vi "red_tweezers_interface.vi"() -> ()   [LabVIEW 2010]
doc: "This is the interface, the one VI which loads all the others. Run this one first.\n\n(the line below ensures settings are saved)\n[Red Tweezers Save Settings]"
uses:
  subvis/line_trapping.ctl
  subvis/spot.ctl
  <vilib>/userDefined/High Color/IMAQdx.ctl
  subvis/mouse_info.ctl
  subvis/selection_element.ctl
  subvis/red_tweezers_globals.vi
  subvis/red_tweezers_globals_INTERNAL_VOLATILE.vi
  <vilib>/Analysis/baseanly.llb/Real A x B.vi
  <vilib>/Analysis/NI_AALBase.lvlib
  <vilib>/vision/driver/NI_Vision_Acquisition_Software.lvlib
panel:
  out "# selected":i16
  out "Last Pattern":T1[](array[typedef]) {"Amplitude Correction" step=0.1; "Line Trapping"."Phase Gradient" step=0.05; "Line Trapping"."Vector"."x" step=1e-06 format="%#_6p"; "Line Trapping"."Vector"."y" step=1e-06 format="%#_6p"; "Line Trapping"."Vector"."z" step=1e-06 format="%#_6p"; "NA Position"."r" step=1e-06; "NA Position"."y" step=1e-06; "NA Position"."x" step=1e-06; "Position"."z" step=1e-06; "Position"."y" step=1e-06; "Position"."x" step=1e-06; "Phase" step=0.7753; "Intensity" step=0.1}
  out "Plugins":T3(array[cluster])=[{"Name"="ASI Stage", "Folder"=path "C:/Users/Richard Bowman/Dropbox/red_tweezers_1_4_rc4/plugins/ASI Stage.llb", "vi reference"=refnum, "Needs to be run"=TRUE, "Error"={"status"=FALSE, "code"=0, "source"=""}}, {"Name"="iTweezers", "Folder"=path "C:/Users/Richard Bowman/Dropbox/red_tweezers_1_4_rc4/plugins/iTweezers.llb", "vi reference"=refnum, "Needs to be run"=TRUE, "Error"={"status"=FALSE, "code"=0, "source"=""}}, {"Name"="MightexLED", "Folder"=path "C:/Users/Richard Bowman/Dropbox/red_tweezers_1_4_rc4/plugins/MightexLED.llb", "vi reference"=refnum, "Needs to be run"=TRUE, "Error"={"status"=FALSE, "code"=0, "source"=""}}]
  in  "Tab":T4(tab)
  out "spots selected":i32=4
  in  "lock aspect ratio":bool=TRUE
  in  "Size":cluster{"x":dbl, "y":dbl, "z":dbl} {"z" step=1e-06 format="%#_4p"; "y" step=1e-06 format="%#_4p"; "x" step=1e-06 format="%#_4p"}
  in  "Position":cluster{"x":dbl, "y":dbl, "z":dbl}={"x"=1e-06, "y"=-6.3e-06, "z"=0.0} {"z" step=1e-06 format="%#_4p"; "y" step=1e-06 format="%#_4p"; "x" step=1e-06 format="%#_4p"}
  in  "phase":dbl step=0.7753
  in  "Vortex Charge":i8
  in  "Intensity":dbl=1.0 step=0.1
  in  "add to selection":bool
  in  "random position":bool
  in  "new spot":bool
  in  "delete":bool
  in  "rotate":bool
  in  "Rotation Axis":u16(ring)=2 items=["Z", "X", "Y", "Custom"]
  in  "Angle (degrees)":dbl=2.0
  in  "Custom Axis":cluster{dbl, dbl, dbl}
  in  "Spot Shape":enum32{"Normal", "Line", "NA", "Mixed"}(tab)=enum."Mixed"
  in  "Line Trapping":T2 {"Phase Gradient" step=0.05; "Vector"."x" step=1e-06 format="%#_4p"; "Vector"."y" step=1e-06 format="%#_4p"; "Vector"."z" step=1e-06 format="%#_4p"}
  in  "Scale back aperture":dbl=1.1 step=0.1
  in  "Scale BA":bool
  in  "Position on back aperture":cluster{"x":dbl, "y":dbl}={"x"=-5.84327907697451e-18, "y"=0.0} {"y" step=0.1 format="%#_4p"; "x" step=0.1 format="%#_4p"}
  in  "Radius on back aperture":dbl=1.1 step=0.1
  in  "Generate":bool
  in  "Pattern":T5(tab)
  in  "Spots across centre":i32=5
  in  "Reference Array?":bool
  in  "Fraction of SLM":dbl=1.0
  in  "Spots across centre":i32=5
  in  "N":cluster{i32, i32}
  in  "spacing/m":dbl=2.0
  in  "Iterations":i32=10
  out "non-uniformity":dbl(slide)=0.031119223416512406 scale=0.0..0.2
  out "efficiency":dbl(slide)=0.8985936267644501 scale=0.0..1.0
  in  "Optimise":bool
  in  "Reset Phase/Amplitude":bool
  in  "Fall-off/m":dbl=0.00025 min=0.0 step=1e-06 format="%#_4p"
  in  "Abort Plugin":bool
  in  "Plugin:":u16(ring)=1 items=["ASI Stage", "iTweezers", "MightexLED"]
  in  "Save Video":bool
  in  "Global ROI (requires restart)":i32[](array[numeric])=[0, 0, 1280, 512]
  in  "Zoom":bool
  in  "Draw ROI":bool
  in  "Zoom to Fit":bool
  out "Image Information":string="640x480 1.93X 8-bit image 255    (0,0)"
  in  "Camera":T6
  out "Video Frame Rate":dbl(knob)=50.00000000000003 scale=0.0..100.0 scale format="%.1f"
  out "Interface Frame Rate":dbl(knob)=97.23240312927678 scale=0.0..100.0 scale format="%.1f"
  in  "stop":bool=TRUE
  out "Image":T7(plugin-control)
  # "The SLM can be used to shape spots; here you can restrict the NA of a spot (so it comes only from part of the back aperture), or create a line-trap"
  # "The traps do not have any spot-shaping applied (so they should just be diffraction-limited focal spots)."
  # "This shapes the amplitude (and phase) of the beam to create extended line traps.  The \"Phase Gradient\" control allows the Poynting vector to push things along the line.  Unfortunately, some work is needed on the scaling factors so the phase gradient control will need tweaking if the line trap has a nonzero z component."
  # "By default,each spot comes from the whole back aperture.  Here, you can limit a spot to come from a specific part of the back aperture."
  # "The control below allows you to scale the whole back aperture (i.e. the position and size of all the apertures).  It's a one-time operation, i.e. only changes things when you push \"ok\"."
  # "A Combination of line-trapping and NA restriction has been applied to these traps.  You can get at the line trap or NA parameters on the other tabs, switching to the NA tab does not delete the line-trap settings."
  # "This tab generates Shack-Hartmann type holograms, which are often useful when aligning the system, and arrays of spots."
  # "The controls above only work when using the \"IMAQdx with ROI Buttons\" case in the bottom loop.  You can save video regardless of camera code though."
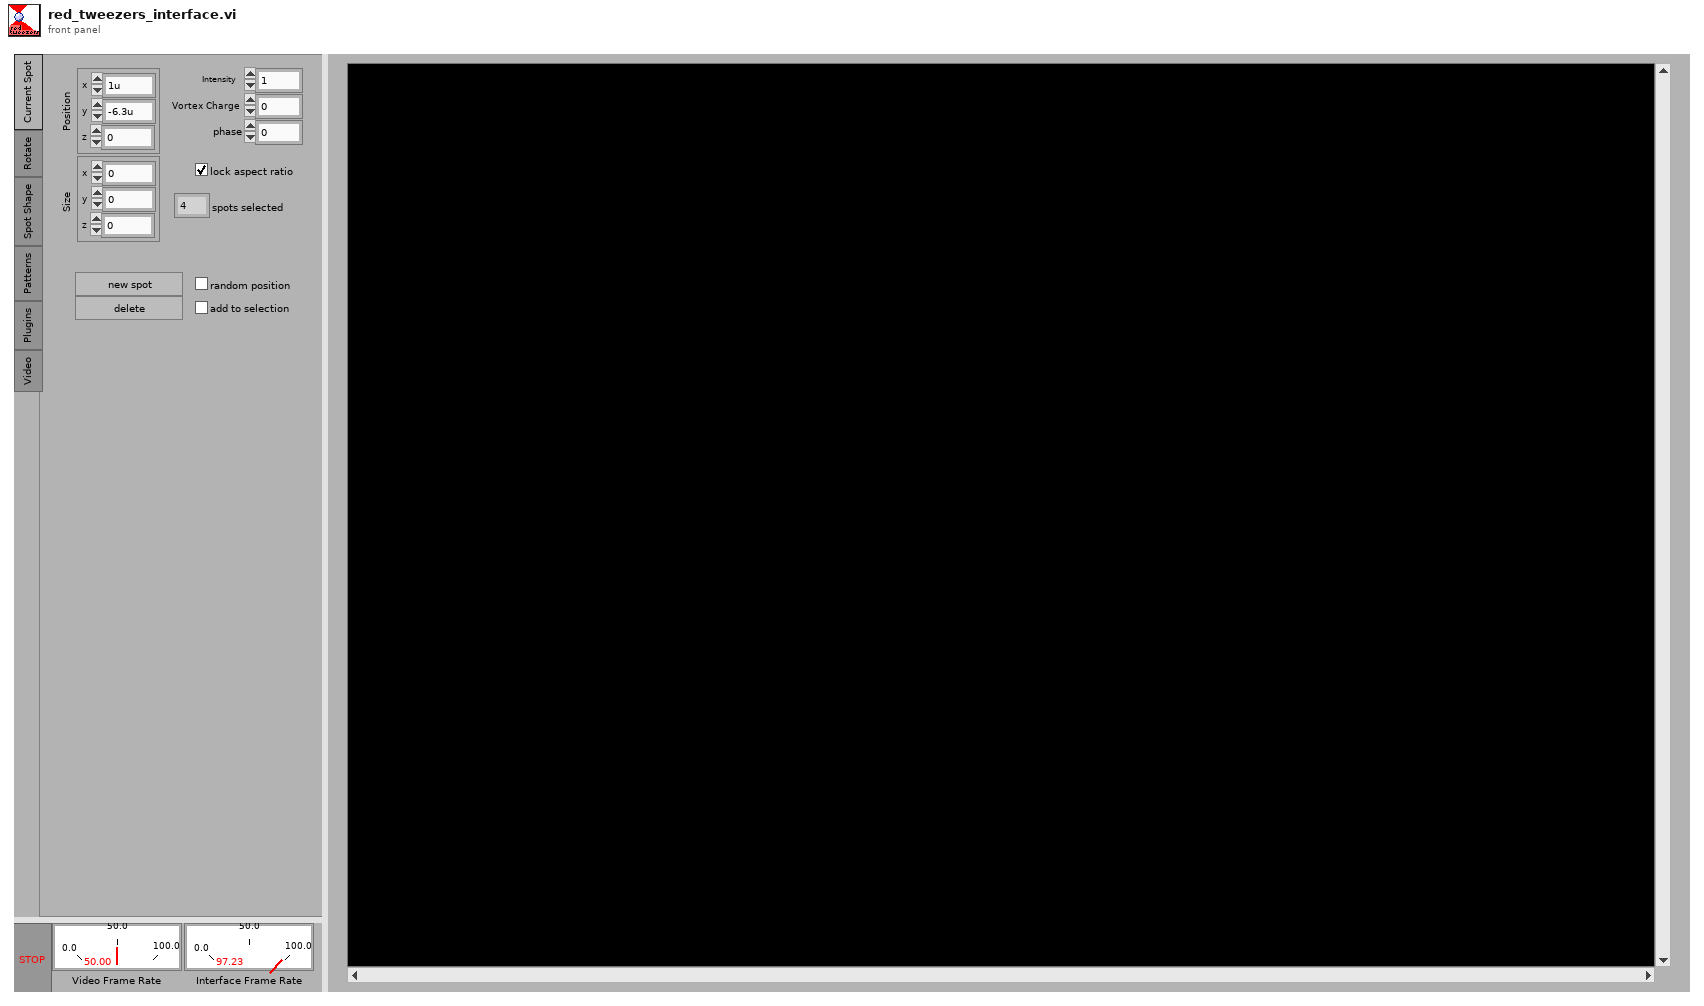
[diagram p1: front panel]
types:
  T1 = typedef "spot.ctl" = cluster{"Position":cluster{"x":dbl, "y":dbl, "z":dbl}, "Intensity":dbl, "Vortex Charge":i8, "Phase":dbl, "NA Position":cluster{"x":dbl, "y":dbl, "r":dbl}, "Line Trapping":T2, "Amplitude Correction":dbl}
  T2 = typedef "line_trapping.ctl" = cluster{"Vector":cluster{"x":dbl, "y":dbl, "z":dbl}, "Phase Gradient":dbl}
  T3 = cluster{"Name":string, "Folder":path, "vi reference":refnum<vi>, "Needs to be run":bool, "Error":errorcluster}[]
  T4 = enum32{"Current Spot", "Rotate", "Spot Shape", "Patterns", "Plugins", "Video"}
  T5 = enum32{"HCP Shack-Hartmann", "Square Shack-Hartmann", "Rectangular Grid"}
  T6 = typedef "IMAQdx.ctl" = refnum<k21>
  T7 = typedef "IMAQ Image.ctl" = refnum<image>
  T8 = typedef "mouse_info.ctl" = cluster{"Button Down":bool, "Dragging":bool, "Position (Image Pixels)":cluster{"X":dbl, "Y":dbl}, "Previous Position (Image Pixels)":cluster{"X":dbl, "Y":dbl}, "Button":u16, "Mods":cluster{"Double Click":bool, "Menu Key":bool}, "PlatMods":cluster{"Shift":bool, "Ctrl":bool, "Alt":bool, "Cmd":bool, "Opt":bool}}
  T9 = typedef "selection_element.ctl" = cluster{"Group ID":i32, "Selected":bool}
  T10 = enum32{"Bad", "Idle", "Run top level", "Running"}
  T11 = cluster{"Average Frame Time":dbl, "millisecond timer value":u32}
  T12 = typedef "Image Type" = u32
  T13 = enum16{"Set guide visibility", "Set grid visibility", "Show front panel", "Render on image"}
  T14 = enum16{"Left Button", "Center Button", "Right Button", "Window Close"}
  T15 = cluster{"number: 0 to 1":dbl, "number: 0 to 1":dbl}
  T16 = typedef "NI_Matrix.lvlib/RealMatrix.ctl" = dbl[][]
  T17 = typedef "overlay_element.ctl" = cluster{"Tool":enum16{"Lines", "Oval", "Rectangle", "Text"}, "Points":cluster{"X":dbl, "Y":dbl}[], "Drawing Mode":u32, "Color":u32, "String":string}
  T18 = enum32{"Current Spot", "Rotate", "Spot Shape", "Patterns", "Plugins", "Video", "Particle Tracking", "Clamping", "Blank"}[]
  T19 = typedef "LVMenuShortCut.ctl" = cluster{"include Shift key?":bool, "include Ctrl key?":bool, "shortcut key":string}
  T20 = typedef "LVPoint32TypeDef.ctl" = cluster{"Horizontal":i32, "Vertical":i32}
  T21 = cluster{"Shift":bool, "Ctrl":bool, "Alt":bool, "Cmd":bool, "Opt":bool}
  T22 = cluster{"Button Down":bool, "Dragging":bool, "Mouse Coords (image pixels)":cluster{dbl, dbl}, "Mouse Coords (image pixels)":cluster{dbl, dbl}, "Button":u16, "Mods":cluster{"Double Click":bool, "Menu Key":bool}, "PlatMods":cluster{"Shift":bool, "Ctrl":bool, "Alt":bool, "Cmd":bool, "Opt":bool}}
  T23 = typedef "AviRefnum.ctl" = refnum<k1>
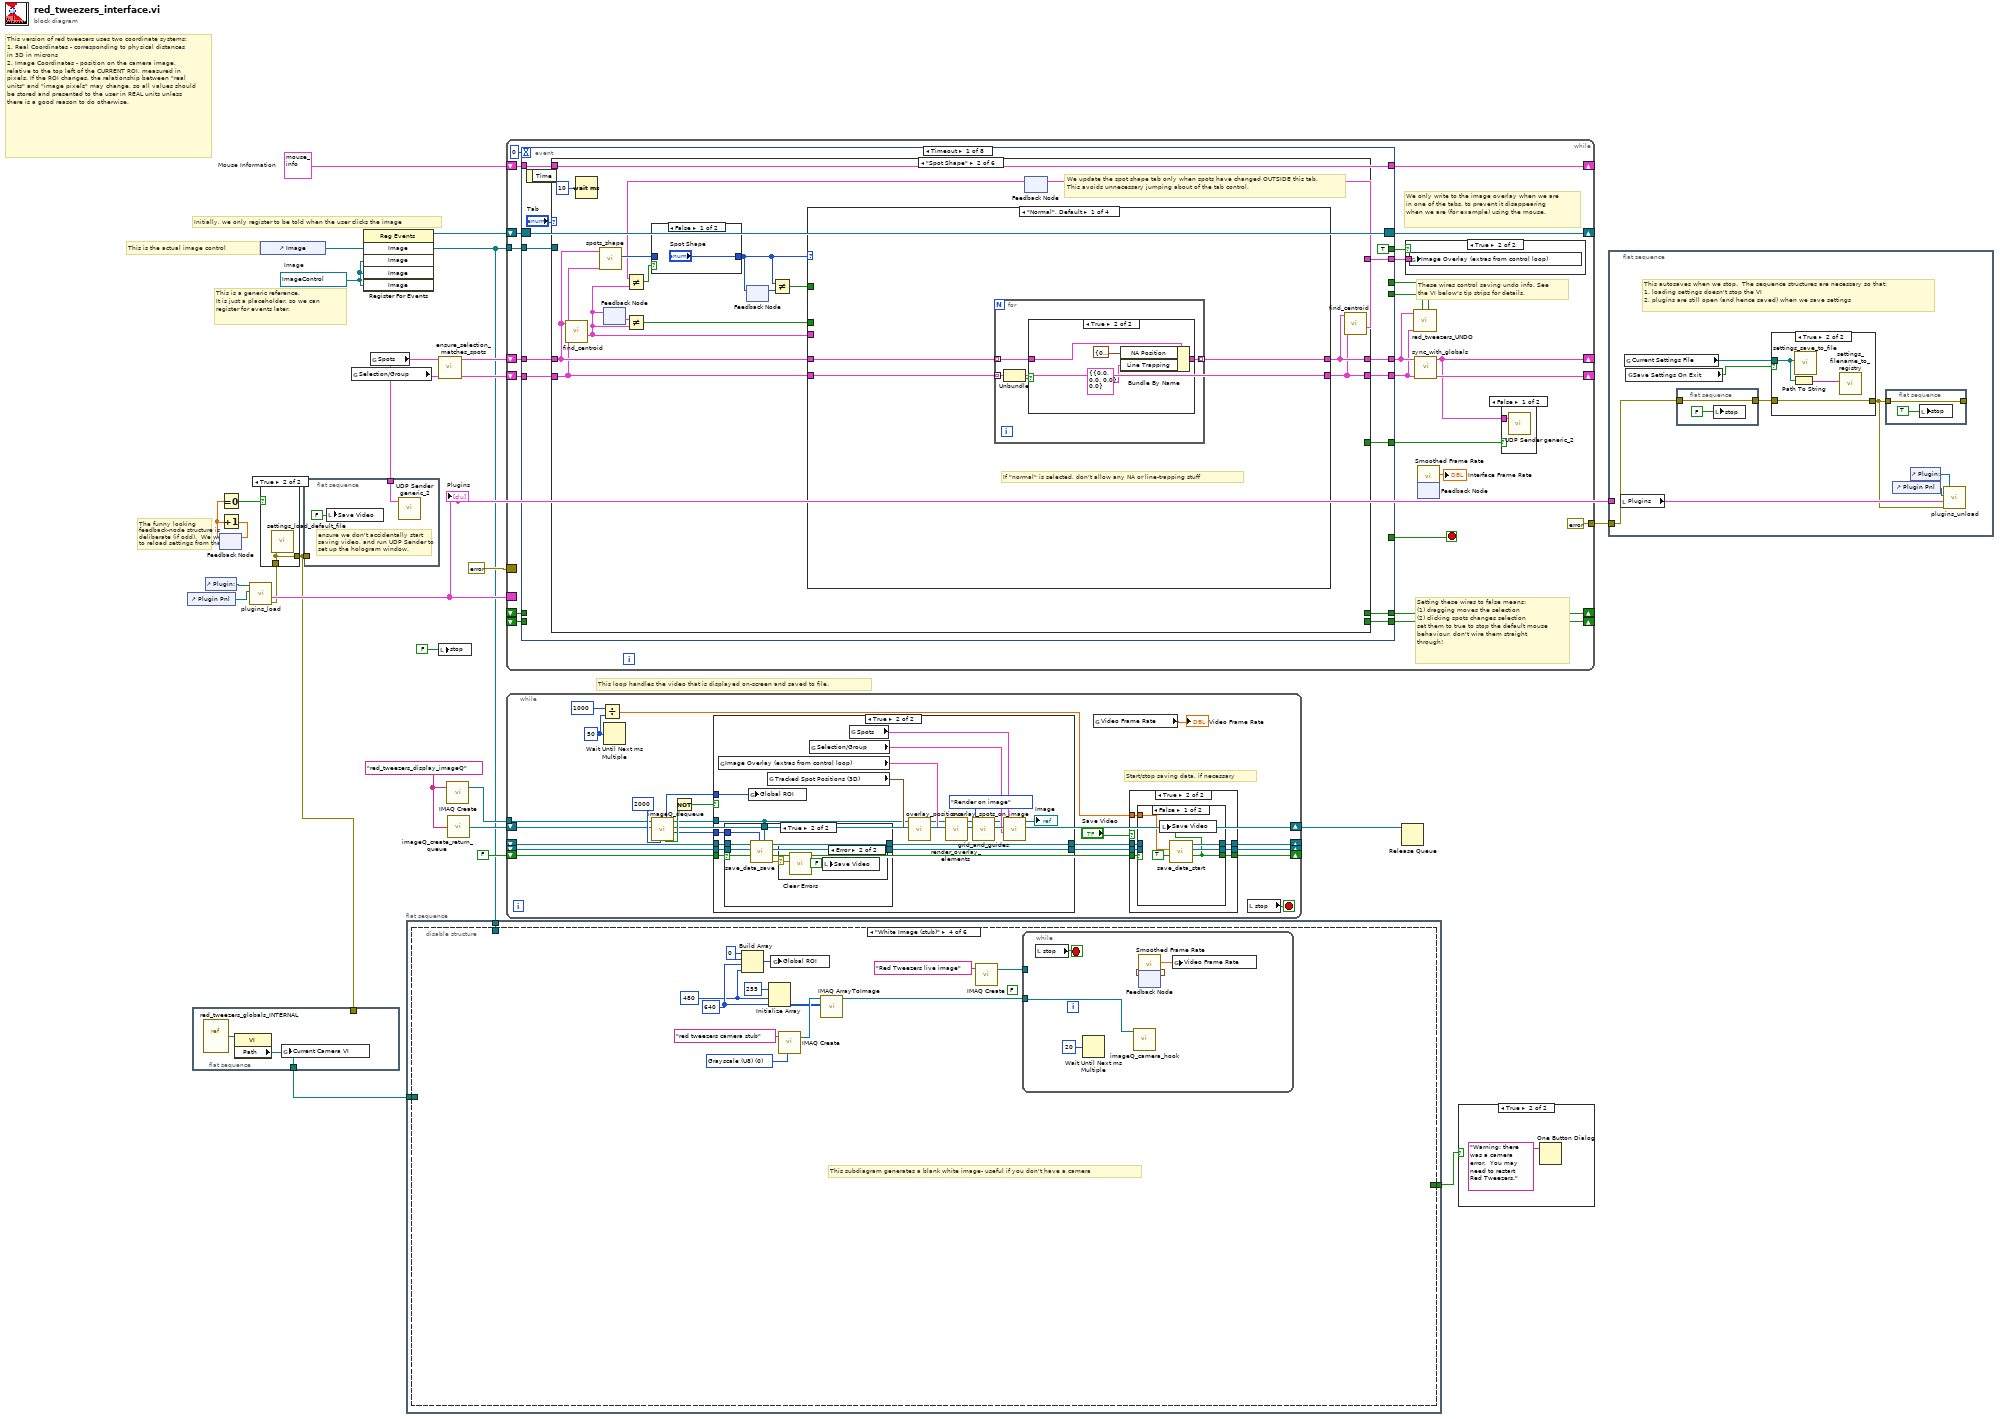
[diagram p0: block diagram]
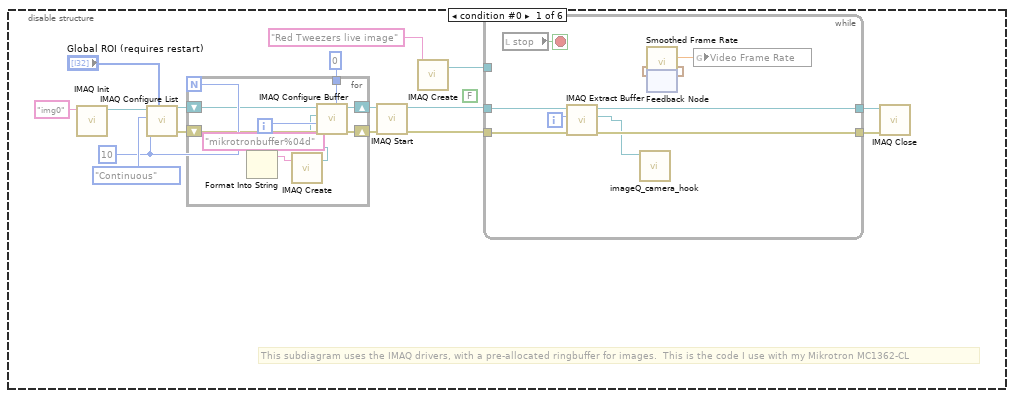
[diagram p3: hidden frame]
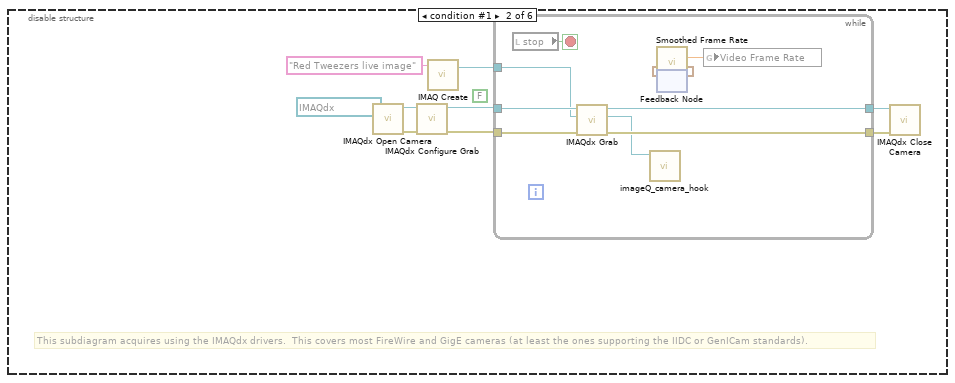
[diagram p4: hidden frame]
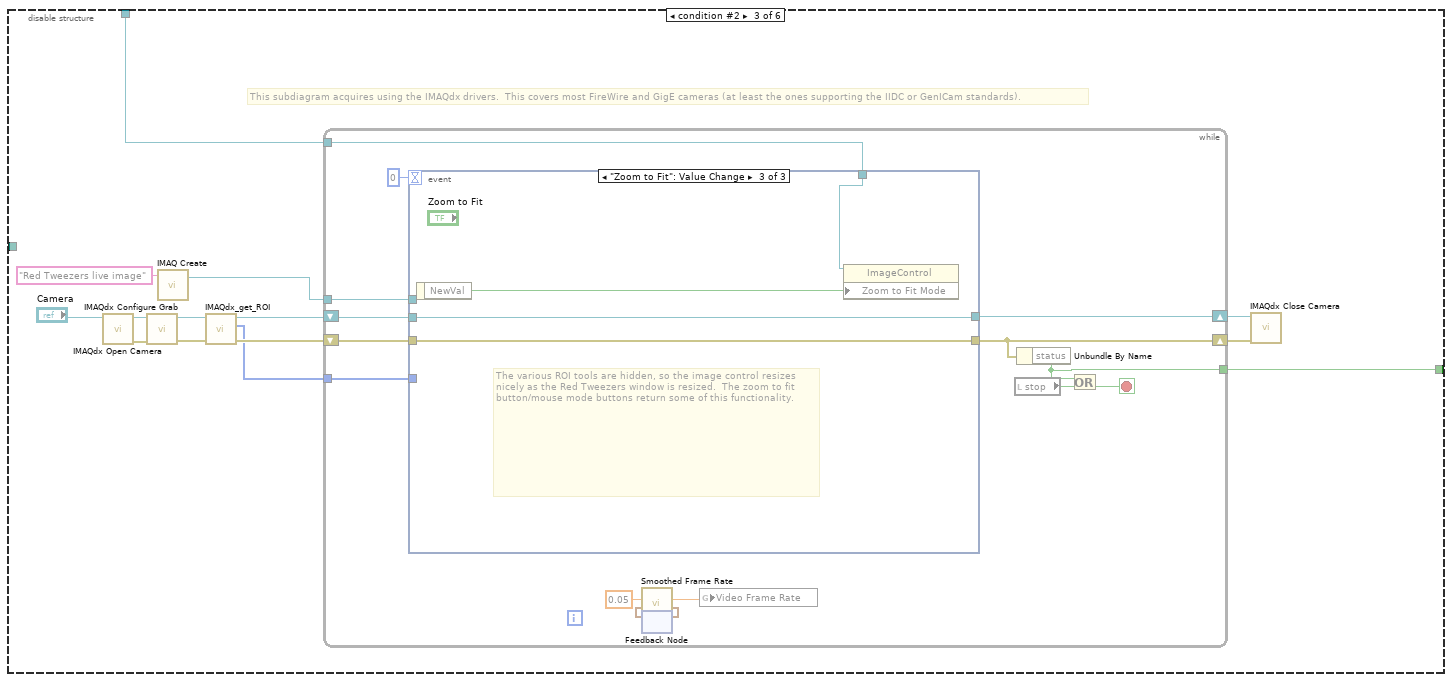
[diagram p5: hidden frame]
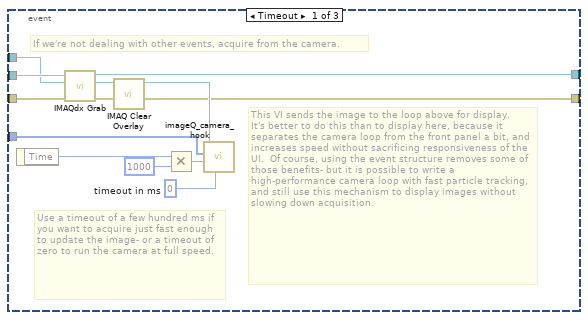
[diagram p6: hidden frame]
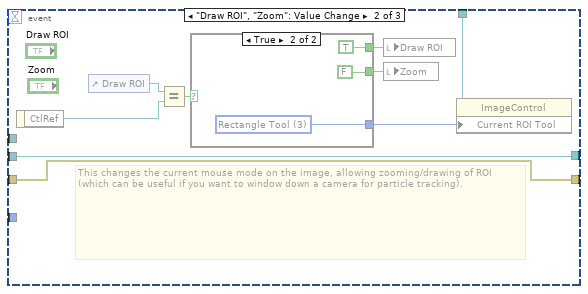
[diagram p7: hidden frame]
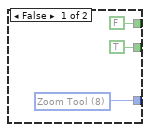
[diagram p8: hidden frame]
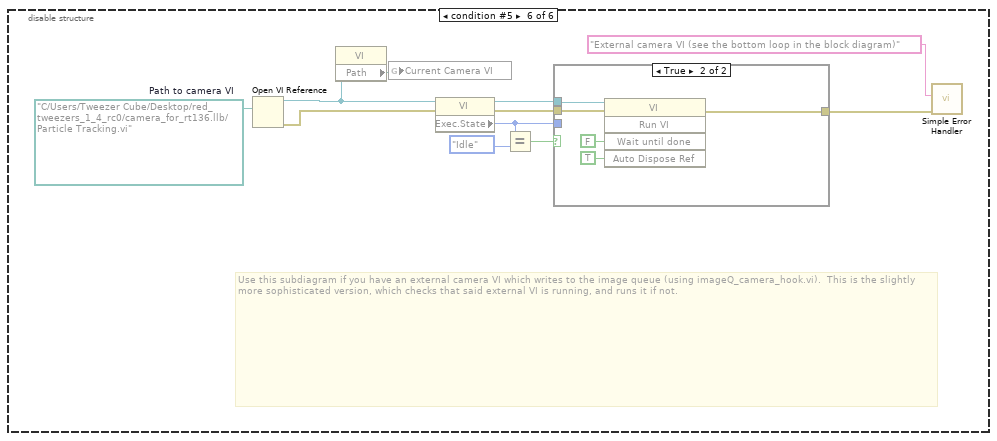
[diagram p10: hidden frame]
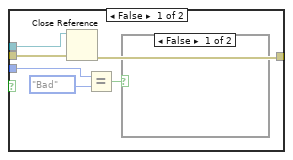
[diagram p11: hidden frame]
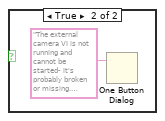
[diagram p12: hidden frame]
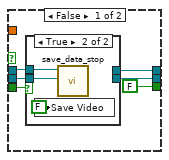
[diagram p13: hidden frame]
diagram:
  w10 = "red_tweezers_display_imageQ" ("Queue Name")
  w22 = T8 {"Button Down"=FALSE, "Dragging"=FALSE, "Position (Image Pixels)"={"X"=0.0, "Y"=0.0}, "Previous Position (Image Pixels)"={"X"=0.0, "Y"=0.0}, "Button"=0, "Mods"={"Double Click"=FALSE, "Menu Key"=FALSE}, "PlatMods"={"Shift"=FALSE, "Ctrl"=FALSE, "Alt"=FALSE, "Cmd"=FALSE, "Opt"=FALSE}}  # Mouse Information
  w23 = refnum<vi> refnum  # Image
  # "The funny looking feedback-node structure is deliberate (if odd).  We want to reload settings from the last used file (stored in the registry) only if this program has not been run since it was last loaded from file/recompiled.  That's why I use an uninitialised shift register: every time the program runs, it increments.  So, if it is zero, this is our first run (or we've been recently recompiled)."
  # "This loop handles the video that is displayed on-screen and saved to file."
  # "Initially, we only register to be told when the user clicks the image"
  # "This is the actual image control"
  # "This is a generic reference.\nIt is just a placeholder, so we can register for events later."
  # "This version of red tweezers uses two coordinate systems: \n1. Real Coordinates - corresponding to physical distances in 3D in microns\n2. Image Coordinates - position on the camera image, relative to the top left of the CURRENT ROI, measured in pixels. If the ROI changes, the relationship between \"real units\" and \"image pixels\" may change, so all values should be stored and presented to the user in REAL units unless there is a good reason to do otherwise."
  n1 = control-ref of="Plugin Pnl"() -> (w19:refnum<vi>)
  n2 = flat-sequence {
    tunnel: [w27] -> w5
    tunnel: w3 -> [_]
    frame #0 {
      n3 = vi-ref "red_tweezers_globals_INTERNAL.vi"() -> (w28:refnum<vi>)
      n4 = property class="VI"(reference=w28) -> ("Path"=w27:path)  [unwired: 1 in, 2 out]
      n5 = global write "red_tweezers_globals_INTERNAL_VOLATILE.vi" "Current Camera VI"(w27) -> ()
    }
  }
  n6 = control-ref of="Plugin:"() -> (w20:refnum<vi>)
  n7 = feedback #1() -> (w13:dbl)  [unwired: 1 in]
  n8 = Equal To 0?(x=w13) -> (x = 0?=w12:bool)
  n9 = Increment(x=w13) -> (x+1=w11:dbl)
  n10 = feedback-in #1(w11) -> ()
  n11 = call "plugins_load.vi"("Sub Panel"=w19, "Plugin Chooser"=w20) -> ("error out"=w14:errorcluster, "Plugins"=w16:T3)  [unwired: 2 in, 2 out]
  "Plugins" <- w16
  n12 = control-ref of="Image"() -> (w4:refnum<vi>)
  n13 = case shown="True" w12 {
    tunnel: w14 -> [_ w29]
    tunnel: [_ w29] -> w3
    frame False {
    }
    frame True {
      n14 = call "settings_load_default_file.vi"("error out"=w29) -> ()
    }
  }
  n15 = flat-sequence {
    tunnel: w3 -> [_]
    tunnel: w2 -> [w31]
    frame #0 {
      # "ensure we don't accidentally start saving video, and run UDP Sender to set up the hologram window."
      n16 = local write "Save Video"(FALSE ("background subtraction")) -> ()
      n17 = call "UDP Sender generic_2.vi"("Spots"=w31) -> ()  [unwired: 2 in, 1 out]
    }
  }
  n18 = global read "red_tweezers_globals.vi" "Selection/Group"() -> (w21:T9[])
  n19 = register-events(w4, w23, w23, w23) -> (reference out=w24:refnum<event-registration>)  [unwired: 2 in, 1 out]
  n20 = global read "red_tweezers_globals.vi" "Spots"() -> (w2:T1[])
  n21 = flat-sequence {
    tunnel: w5 -> [w34]
    tunnel: w4 -> [w33]
    tunnel: [w32] -> w1
    frame #0 {
      n22 = disable-structure shown="\"White Image (stub)\"" {
        disable-tunnel: w34 -> [_ _ _ _ _ _]
        disable-tunnel: w33 -> [_ _ w92 _ _ _]
        disable-tunnel: [_ _ w91 _ _ _] -> w32
        frame condition #0 {
          w36 = u32 10 ("Number of buffers")
          (unwired) FALSE ("background subtraction")
          # "This subdiagram uses the IMAQ drivers, with a pre-allocated ringbuffer for images.  This is the code I use with my Mikrotron MC1362-CL"
          n23 = call <vilib>:"IMAQ Init.vi"("Interface Name"="img0") -> ("IMAQ Session Out"=w43:refnum<k11>)  [unwired: 9 in, 1 out]
          n24 = call <vilib>:"IMAQ Configure List.vi"("Region of interest"="Global ROI (requires restart)", "Number of buffers"=w36, "Continuous?"=enum16{"One-Shot", "Continuous"}."Continuous", "IMAQ Session In"=w43) -> ("error out"=w37:errorcluster, "IMAQ Session Out"=w39:refnum<k11>)  [unwired: 6 in]
          n25 = for {
            N: w36 -> [_]
            tunnel: 0 ("Channel") -> [w56]
            shift-right: [w59] -> w41
            shift-left: w37 -> [w55]
            shift-right: [w58] -> w40
            shift-left: w39 -> [w57]
            i -> [w54]
            n26 = Format Into String(format string="mikrotronbuffer%04d", w54) -> (resulting string=w52:string)  [unwired: 2 in, 1 out]
            n27 = call "IMAQ Create"("Image Name"=w52) -> ("New Image"=w51:T7)  [unwired: 4 in, 1 out]
            n28 = call <vilib>:"IMAQ Configure Buffer.vi"("Channel"=w56, "error in (no error)"=w55, "Buffer Number"=w54, "Image In"=w51, "IMAQ Session In"=w57) -> ("error out"=w59:errorcluster, "IMAQ Session Out"=w58:refnum<k11>)  [unwired: 5 in]
          }
          n29 = call <vilib>:"IMAQ Start.vi"("error in (no error)"=w41, "IMAQ Session In"=w40) -> ("error out"=w47:errorcluster, "IMAQ Session Out"=w48:refnum<k11>)  [unwired: 8 in]
          n30 = call "IMAQ Create"("Image Name"="Red Tweezers live image") -> ("New Image"=w49:T7)  [unwired: 3 in, 2 out]
          n31 = while {
            tunnel: w48 -> [w67]
            tunnel: w47 -> [w66]
            tunnel: w49 -> [_]
            tunnel: [w68] -> w45
            tunnel: [w61] -> w46
            i -> [w63]
            stop <- w69 stop-if-true
            n32 = local read "stop"() -> (w69:bool)
            n33 = call <vilib>:"IMAQ Extract Buffer.vi"("error in (no error)"=w66, "Buffer to extract"=w63, "IMAQ Session In"=w67) -> ("error out"=w61:errorcluster, "Image Out"=w60:T7, "IMAQ Session Out"=w68:refnum<k11>)  [unwired: 3 in, 3 out]
            n34 = call "imageQ_camera_hook.vi"("Image"=w60) -> ()  [unwired: 11 in]
            n35 = feedback #2() -> (w64:T11)  [unwired: 1 in]
            n36 = call "Smoothed Frame Rate.vi"("Feedback In"=w64) -> ("Feedback Out"=w65:T11, "Frame Rate"=w62:dbl)  [unwired: 1 in, 4 out]
            n37 = feedback-in #2(w65) -> ()
            n38 = global write "red_tweezers_globals_INTERNAL_VOLATILE.vi" "Video Frame Rate"(w62) -> ()
          }
          n39 = call <vilib>:"IMAQ Close.vi"("error in (no error)"=w46, "IMAQ Session In"=w45) -> ()  [unwired: 9 in, 1 out]
        }
        frame condition #1 {
          (unwired) FALSE ("background subtraction")
          # "This subdiagram acquires using the IMAQdx drivers.  This covers most FireWire and GigE cameras (at least the ones supporting the IIDC or GenICam standards)."
          n40 = call <vilib>:"IMAQdx Open Camera.vi"("Session In"=T6 "dalsaGenie") -> ("error out"=w72:errorcluster, "Session Out"=w71:T6)  [unwired: 9 in]
          n41 = call <vilib>:"IMAQdx Configure Grab.vi"("error in"=w72, "Session In"=w71) -> ("error out"=w73:errorcluster, "Session Out"=w74:T6)  [unwired: 8 in]
          n42 = call "IMAQ Create"("Image Name"="Red Tweezers live image") -> ("New Image"=w77:T7)  [unwired: 3 in, 2 out]
          n43 = while {
            tunnel: w74 -> [w86]
            tunnel: w73 -> [w85]
            tunnel: w77 -> [w79]
            tunnel: [w87] -> w75
            tunnel: [w81] -> w76
            stop <- w88 stop-if-true
            n44 = local read "stop"() -> (w88:bool)
            n45 = call <vilib>:"IMAQdx Grab.vi"("error in"=w85, "Image In"=w79, "Session In"=w86) -> ("error out"=w81:errorcluster, "Image Out"=w80:T7, "Session Out"=w87:T6)  [unwired: 5 in, 1 out]
            n46 = call "imageQ_camera_hook.vi"("Image"=w80) -> ()  [unwired: 11 in]
            n47 = feedback #3() -> (w83:T11)  [unwired: 1 in]
            n48 = call "Smoothed Frame Rate.vi"("Feedback In"=w83) -> ("Feedback Out"=w84:T11, "Frame Rate"=w82:dbl)  [unwired: 1 in, 4 out]
            n49 = feedback-in #3(w84) -> ()
            n50 = global write "red_tweezers_globals_INTERNAL_VOLATILE.vi" "Video Frame Rate"(w82) -> ()
          }
          n51 = call <vilib>:"IMAQdx Close Camera.vi"("error in"=w76, "Session In"=w75) -> ()  [unwired: 9 in, 1 out]
        }
        frame condition #2 {
          # "This subdiagram acquires using the IMAQdx drivers.  This covers most FireWire and GigE cameras (at least the ones supporting the IIDC or GenICam standards)."
          n52 = call <vilib>:"IMAQdx Open Camera.vi"("Session In"="Camera") -> ("error out"=w100:errorcluster, "Session Out"=w99:T6)  [unwired: 9 in]
          n53 = call <vilib>:"IMAQdx Configure Grab.vi"("error in"=w100, "Session In"=w99) -> ("error out"=w96:errorcluster, "Session Out"=w97:T6)  [unwired: 8 in]
          n54 = call "IMAQ Create"("Image Name"="Red Tweezers live image") -> ("New Image"=w94:T7)  [unwired: 3 in, 2 out]
          n55 = call "IMAQdx_get_ROI.vi"("Session In"=w97) -> ("ROI"=w93:u32[], "Session Out"=w95:T6)  [unwired: 8 in]
          n56 = while {
            shift-right: [w109] -> w89
            shift-left: w96 -> [w110]
            shift-right: [w106] -> w90
            shift-left: w95 -> [w107]
            tunnel: w94 -> [w105]
            tunnel: w93 -> [w104]
            tunnel: w92 -> [w103]
            tunnel: [w102] -> w91
            stop <- w116 stop-if-true
            n57 = event shown="[2] \"Zoom to Fit\": Value Change" {
              selector: _ -> [_ _ _]
              dyn-events: _ -> [_ _ _]
              timeout: 0 -> [_ _ _]
              tunnel: w110 -> [w123 w130 w145]
              tunnel: [w122 w130 w145] -> w109
              tunnel: w107 -> [w121 w131 w146]
              tunnel: [w120 w131 w146] -> w106
              tunnel: w105 -> [w119 _ _]
              tunnel: w104 -> [w118 _ _]
              tunnel: w103 -> [_ w129 w144]
              event Timeout {
                w117 = 0  # timeout in ms
                # "Use a timeout of a few hundred ms if you want to acquire just fast enough to update the image- or a timeout of zero to run the camera at full speed."
                # "This VI sends the image to the loop above for display.\nIt's better to do this than to display here, because it separates the camera loop from the front panel a bit, and increases speed without sacrificing responsiveness of the UI.  Of course, using the event structure removes some of those benefits- but it is possible to write a high-performance camera loop with fast particle tracking, and still use this mechanism to display images without slowing down acquisition."
                # "If we're not dealing with other events, acquire from the camera."
                n58 = event-data() -> ("Time"=w128:u32)  [unwired: 1 in]
                n59 = call <vilib>:"IMAQdx Grab.vi"("error in"=w123, "Image In"=w119, "Session In"=w121) -> ("error out"=w122:errorcluster, "Image Out"=w125:T7, "Session Out"=w120:T6)  [unwired: 5 in, 1 out]
                n60 = call "IMAQ Clear Overlay"("Image"=w125) -> ("Image Out"=w124:T7)  [unwired: 9 in, 1 out]
                n61 = Multiply(x=w128, y=u32 1000) -> (x*y=w126:u32)
                n62 = call "imageQ_camera_hook.vi"("timeout in ms (0=don't wait if there are no requests)"=w117, "Timestamp/us"=w126, "ROI"=w118, "Image"=w124) -> ()  [unwired: 8 in]
              }
              event "Draw ROI", "Zoom": Value Change {
                # "This changes the current mouse mode on the image, allowing zooming/drawing of ROI (which can be useful if you want to window down a camera for particle tracking)."
                n63 = event-data() -> ("CtlRef"=w136:refnum<vi>)  [unwired: 1 in]
                n64 = control-ref of="Draw ROI"() -> (w137:refnum<vi>)
                n65 = Equal?(x=w137, y=w136) -> (x = y?=w135:bool)
                n66 = case shown="True" w135 {
                  tunnel: [w140 w143] -> w134
                  tunnel: [TRUE ("stop") FALSE ("stop")] -> w132
                  tunnel: [FALSE ("Update Indicators?") TRUE ("Update Indicators?")] -> w133
                  frame False {
                    w140 = u32 8 items=["Zoom Tool"=8, "Selection Tool"=0, "Pan Tool"=9, "Point Tool"=1, "Line Tool"=2, "Rectangle Tool"=3, "Rotated Rectangle Tool"=12, "Polyline Tool"=10, "Polygon Tool"=5, "Freehand Tool"=11, "Closed Freehand Tool"=6, "Ellipse Tool"=4, "Annulus Tool"=7] ("Current ROI Tool")
                  }
                  frame True {
                    w143 = u32 3 items=["Zoom Tool"=8, "Selection Tool"=0, "Pan Tool"=9, "Point Tool"=1, "Line Tool"=2, "Rectangle Tool"=3, "Rotated Rectangle Tool"=12, "Polyline Tool"=10, "Polygon Tool"=5, "Freehand Tool"=11, "Closed Freehand Tool"=6, "Ellipse Tool"=4, "Annulus Tool"=7] ("Current ROI Tool")
                  }
                }
                n67 = local write "Draw ROI"(w133) -> ()
                n68 = local write "Zoom"(w132) -> ()
                n69 = property on="Property Node" class="ImageControl"(reference=w129, "Current ROI Tool"=w134) -> ()  [unwired: 1 in, 2 out]
              }
              event "Zoom to Fit": Value Change {
                # "The various ROI tools are hidden, so the image control resizes nicely as the Red Tweezers window is resized.  The zoom to fit button/mouse mode buttons return some of this functionality."
                n70 = event-data() -> ("NewVal"=w147:bool)  [unwired: 1 in]
                n71 = property on="Property Node" class="ImageControl"(reference=w144, "Zoom to Fit Mode"=w147) -> ()  [unwired: 1 in, 2 out]
              }
            }
            n72 = feedback #4() -> (w115:T11)  [unwired: 1 in]
            n73 = call "Smoothed Frame Rate.vi"("Feedback In"=w115, "Alpha"=0.05) -> ("Feedback Out"=w114:T11, "Frame Rate"=w111:dbl)  [unwired: 4 out]
            n74 = feedback-in #4(w114) -> ()
            n75 = global write "red_tweezers_globals_INTERNAL_VOLATILE.vi" "Video Frame Rate"(w111) -> ()
            n76 = local read "stop"() -> (w112:bool)
            n77 = Unbundle By Name(w109) -> ("status"=w102:bool)
            n78 = Or(x=w102, y=w112) -> (x .or. y?=w116:bool)
          }
          n79 = call <vilib>:"IMAQdx Close Camera.vi"("error in"=w89, "Session In"=w90) -> ()  [unwired: 9 in, 1 out]
        }
        frame condition #3 (active) {
          w149 = 0 ("element")
          w151 = 640 ("dimension size")
          w150 = 480 ("dimension size")
          w152 = T12 0 items=["Grayscale (U8)", "Grayscale (I16)", "Grayscale (SGL)", "Complex (CSG)", "RGB (U32)", "HSL (U32)", "RGB (U64)", "Grayscale (U16)"] ("Image Type")
          (unwired) FALSE ("background subtraction")
          # "This subdiagram generates a blank white image- useful if you don't have a camera"
          n80 = Build Array(w149, w149, w151, w150) -> (w148:i32[])
          n81 = Initialize Array(u8 255 ("element"), w150, w151) -> (w153:u8[][])
          n82 = global write "red_tweezers_globals_INTERNAL.vi" "Global ROI"(w148) -> ()
          n83 = call "IMAQ Create"("Image Name"="red tweezers camera stub", "Image Type"=w152) -> ("New Image"=w154:T7)  [unwired: 2 in, 2 out]
          n84 = call "IMAQ ArrayToImage"("Image Pixels (U8)"=w153, "Image"=w154) -> ("Image Out"=w157:T7)  [unwired: 8 in, 1 out]
          n85 = call "IMAQ Create"("Image Name"="Red Tweezers live image") -> ("New Image"=w158:T7)  [unwired: 3 in, 2 out]
          n86 = while {
            tunnel: w157 -> [w161]
            tunnel: w158 -> [_]
            stop <- w165 stop-if-true
            n87 = local read "stop"() -> (w165:bool)
            n88 = Wait Until Next ms Multiple(millisecond multiple=u32 20) -> ()  [unwired: 1 out]
            n89 = call "imageQ_camera_hook.vi"("Image"=w161) -> ()  [unwired: 11 in]
            n90 = feedback #5() -> (w163:T11)  [unwired: 1 in]
            n91 = call "Smoothed Frame Rate.vi"("Feedback In"=w163) -> ("Feedback Out"=w164:T11, "Frame Rate"=w162:dbl)  [unwired: 1 in, 4 out]
            n92 = feedback-in #5(w164) -> ()
            n93 = global write "red_tweezers_globals_INTERNAL_VOLATILE.vi" "Video Frame Rate"(w162) -> ()
          }
        }
        frame condition #4 {
          # "Use this subdiagram if you have an external camera VI which writes to the image queue (using imageQ_camera_hook.vi)"
        }
        frame condition #5 {
          w166 = path "C:/Users/Tweezer Cube/Desktop/red_tweezers_1_4_rc0/camera_for_rt136.llb/Particle Tracking.vi"  # Path to camera VI
          # "Use this subdiagram if you have an external camera VI which writes to the image queue (using imageQ_camera_hook.vi).  This is the slightly more sophisticated version, which checks that said external VI is running, and runs it if not."
          n94 = Open VI Reference(vi path=w166) -> (vi reference=w167:refnum<vi>, error out=w169:errorcluster)  [unwired: 5 in]
          n95 = property class="VI"(reference=w167) -> ("Path"=w168:path)  [unwired: 1 in, 2 out]
          n96 = global write "red_tweezers_globals_INTERNAL_VOLATILE.vi" "Current Camera VI"(w168) -> ()
          n97 = property class="VI"(reference=w167, error in=w169) -> (reference out=w174:refnum<vi>, error out=w173:errorcluster, "Exec.State"=w171:T10)
          n98 = Equal?(x=w171, y=T10."Idle") -> (x = y?=w175:bool)
          n99 = case shown="True" w175 {
            tunnel: w174 -> [w179 w188]
            tunnel: w173 -> [w178 w185]
            tunnel: [w177 w184] -> w170
            tunnel: w171 -> [w181 _]
            frame False {
              n100 = Close Reference(reference=w179, error in (no error)=w178) -> (error out=w177:errorcluster)
              n101 = Equal?(x=w181, y=T10."Bad") -> (x = y?=w180:bool)
              n102 = case shown="False" w180 {
                frame False {
                }
                frame True {
                  n103 = One Button Dialog(message="The external camera VI is not running and cannot be started- it's probably broken or missing.  Check the static/dynamically loaded VI reference in the bottom loop on the block diagram.") -> ()  [unwired: 1 in, 1 out]
                }
              }
            }
            frame True {
              n104 = invoke class="VI" method="Run VI"(reference=w188, error in=w185, "Wait until done"=FALSE ("Wait Until Done"), "Auto Dispose Ref"=TRUE ("Auto Dispose Reference")) -> (error out=w184:errorcluster)  [unwired: 1 in, 4 out]
            }
          }
          n105 = call <vilib>:"Simple Error Handler.vi"("error source (\" \")"="External camera VI (see the bottom loop in the block diagram)" ("error source (\" \")"), "error in (no error)"=w170) -> ()  [unwired: 3 in, 5 out]
        }
      }
    }
  }
  n106 = local write "stop"(FALSE ("STOP")) -> ()
  n107 = call "ensure_selection_matches_spots.vi"("Selection and Groups in"=w21, "Spots"=w2) -> ("Selection and Groups out"=w26:T9[], "Spots (duplicate)"=w25:T1[])  [unwired: 4 in]
  n108 = call "IMAQ Create"("Image Name"=w10) -> ("New Image"=w8:T7)  [unwired: 4 in, 1 out]
  n109 = call "imageQ_create_return_queue.vi"("Queue Name"=w10) -> ("queue out"=w9:refnum<queue>)
  n110 = while {
    shift-right: [w190] -> _
    shift-left: w25 -> [w209]
    shift-right: [w208] -> _
    shift-left: w26 -> [w207]
    shift-right: [w211] -> _
    shift-left: _ -> [w202]
    shift-right: [w210] -> _
    shift-left: _ -> [w201]
    tunnel: w4 -> [w206]
    shift-right: [w200] -> _
    shift-left: w22 -> [w199]
    shift-right: [w203] -> _
    shift-left: w24 -> [w204]
    border: errorcluster {"status"=FALSE, "code"=0, "source"=""} ("error out") -> [_]
    tunnel: [errorcluster {"status"=FALSE, "code"=0, "source"=""} ("error in (no error)")] -> w17
    border: w16 -> [_]
    stop <- w191 stop-if-true
    # "We only write to the image overlay when we are in one of the tabs, to prevent it disappearing when we are (for example) using the mouse."
    # "These wires control saving undo info. See the VI below's tip strips for details."
    # "Setting these wires to false means:\n(1) dragging moves the selection\n(2) clicking spots changes selection\nset them to true to stop the default mouse behaviour, don't wire them straight through!"
    n111 = event shown="[0] Timeout" {
      selector: w204 -> [w220 w815 w820 w1041 w1069 w1086 w1176 _]
      dyn-events: [w220 w814 w820 w1039 w1066 w1087 w1176 _] -> w203
      timeout: 0 -> [_ _ _ _ _ _ _ _]
      tunnel: [w228 _ w822 w1036 w1071 w1077 w1162 _] -> w211
      tunnel: [w227 _ w821 w1035 w1070 w1076 w1166 _] -> w210
      tunnel: [w226 _ _ _ _ _ _ _] -> w189
      tunnel: w209 -> [w225 w810 w827 w1031 w1064 w1083 w1171 w1247]
      tunnel: [w224 w810 w825 w1031 w1064 w1072 w1169 w1247] -> w197
      tunnel: [w223 w809 w824 w1030 w1063 w1084 w1168 w1246] -> w196
      tunnel: w207 -> [w222 w809 w826 w1030 w1063 w1082 w1170 w1246]
      tunnel: w206 -> [w221 w811 w817 w1029 w1067 w1085 w1172 _]
      tunnel: [w219 _ w819 w1040 T8 {"Button Down"=FALSE, "Dragging"=FALSE, "Position (Image Pixels)"={"X"=0.0, "Y"=0.0}, "Previous Position (Image Pixels)"={"X"=0.0, "Y"=0.0}, "Button"=0, "Mods"={"Double Click"=FALSE, "Menu Key"=FALSE}, "PlatMods"={"Shift"=FALSE, "Ctrl"=FALSE, "Alt"=FALSE, "Cmd"=FALSE, "Opt"=FALSE}} T8 {"Button Down"=FALSE, "Dragging"=FALSE, "Position (Image Pixels)"={"X"=0.0, "Y"=0.0}, "Previous Position (Image Pixels)"={"X"=0.0, "Y"=0.0}, "Button"=0, "Mods"={"Double Click"=FALSE, "Menu Key"=FALSE}, "PlatMods"={"Shift"=FALSE, "Ctrl"=FALSE, "Alt"=FALSE, "Cmd"=FALSE, "Opt"=FALSE}} w1175 _] -> w200
      tunnel: w199 -> [w219 _ w819 _ _ w1081 w1165 _]
      tunnel: w202 -> [_ _ w822 w1036 w1071 w1077 w1162 _]
      tunnel: w201 -> [_ _ w821 w1035 w1070 w1076 w1166 _]
      tunnel: [w218 _ _ _ _ _ _ _] -> w198
      tunnel: [_ _ w818 _ _ _ TRUE _] -> w195
      tunnel: [_ _ _ TRUE TRUE TRUE FALSE _] -> w194
      tunnel: [TRUE _ _ _ _ _ _ _] -> w192
      tunnel: [_ _ _ _ _ _ _ "stop"] -> w191
      event Timeout {
        n112 = event-data() -> ()  [unwired: 1 in, 1 out]
        n113 = case shown="\"Spot Shape\"" "Tab" {
          tunnel: [w243 w435 w582 w684 w765 w803] -> w224
          tunnel: w225 -> [w240 w437 w583 w686 w765 w803]
          tunnel: w222 -> [w239 w436 w580 w685 w764 w802]
          tunnel: [w242 w434 w581 w683 w764 w802] -> w223
          tunnel: [w229 _ TRUE _ _ _] -> w228
          tunnel: [w229 _ _ _ _ _] -> w227
          tunnel: [_ _ _ FALSE _ _] -> w226
          tunnel: w221 -> [_ _ _ _ _ w799]
          tunnel: w219 -> [_ _ w562 _ _ _]
          tunnel: [_ _ w564 _ _ _] -> w218
          frame "Current Spot", Default {
            w229 = FALSE
            # "If it's out of date, update front panel"
            n114 = call "find_centroid.vi"("Selection and Groups"=w239, "Spots"=w240) -> ("Mean Values"=w237:T1, "size"=w231:cluster{"x":dbl, "y":dbl, "z":dbl}, "centroid"=w232:cluster{"x":dbl, "y":dbl, "z":dbl}, "# selected"=→"spots selected":i16)  [unwired: 2 in, 1 out]
            n115 = feedback-in #6(w237) -> ()
            n116 = feedback #6() -> (w238:T1)  [unwired: 1 in]
            n117 = feedback #7() -> (w236:cluster{"x":dbl, "y":dbl, "z":dbl})  [unwired: 1 in]
            n118 = feedback-in #7(w231) -> ()
            n119 = Not Equal?(x=w238, y=w237) -> (x != y?=w235:bool)
            n120 = Not Equal?(x=w236, y=w231) -> (x != y?=w234:bool)
            n121 = Or(x=w235, y=w234) -> (x .or. y?=w233:bool)
            n122 = case shown="True" w233 {
              tunnel: w237 -> [_ w249]
              tunnel: w231 -> [_ w244]
              frame False {
              }
              frame True {
                n123 = Unbundle By Name(w249) -> ("Position"=w245:cluster{"x":dbl, "y":dbl, "z":dbl}, "Intensity"=w247:dbl, "Vortex Charge"=w246:i8, "Phase"=w248:dbl)
                n124 = local write "Size"(w244) -> ()
                n125 = local write "Vortex Charge"(w246) -> ()
                n126 = local write "Intensity"(w247) -> ()
                n127 = local write "Position"(w245) -> ()
                n128 = local write "phase"(w248) -> ()
              }
            }
            n129 = event shown="[2] \"new spot\": Value Change" {
              selector: _ -> [_ _ _ _ _ _ _ _]
              dyn-events: _ -> [_ _ _ _ _ _ _ _]
              timeout: 10 -> [_ _ _ _ _ _ _ _]
              tunnel: w240 -> [w251 w255 w269 w296 w322 w367 w393 w416]
              tunnel: w239 -> [w250 w254 w272 w294 w309 w364 w390 w414]
              tunnel: [w251 w253 w270 w295 w310 w365 w391 w415] -> w243
              tunnel: [w250 w252 w271 w294 w309 w364 w390 w414] -> w242
              tunnel: w232 -> [_ _ _ _ w321 _ _ _]
              event Timeout {
                n130 = event-data() -> ()  [unwired: 3 out]
              }
              event "delete": Value Change {
                n131 = event-data() -> ()  [unwired: 7 out]
                n132 = call "delete_selected_spots.vi"("Selection/Group 3"=w254, "Spots 3"=w255) -> ("Selection/Group 2"=w252:T9[], "Spots 2"=w253:T1[])  [unwired: 4 in]
              }
              event "new spot": Value Change {
                # "If we're not adding it to the selection, de-select all the other spots"
                n133 = event-data() -> ()  [unwired: 7 out]
                n134 = call "coords_ROI_currentimage.vi"() -> ("Mono ROI"=w256:i32[])
                n135 = case shown="False" "add to selection" {
                  tunnel: w272 -> [w285 w290]
                  tunnel: [w284 w290] -> w267
                  frame False {
                    n136 = for {
                      tunnel: w285 -> [w288] mode=indexing
                      tunnel: [w289] -> w284 mode=indexing
                      n137 = Unbundle(w288) -> ("Group ID"=w287:i32)  [unwired: 1 out]
                      n138 = Bundle(cluster=w288, "Group ID"=w287, "Selected"=FALSE ("Label.Visible")) -> (w289:T9)
                    }
                  }
                  frame True {
                  }
                }
                n139 = Index Array(array=w256) -> (element #1=w262:i32, element #2=w263:i32, element #3=w261:i32, element #4=w260:i32)  [unwired: 4 in]
                n140 = Bundle("Numeric"=w262, "Numeric"=w263) -> (w257:cluster{"Numeric":i32, "Numeric":i32})  [unwired: 1 in]
                n141 = Bundle("Numeric"=w261, "Numeric"=w260) -> (w259:cluster{"Numeric":i32, "Numeric":i32})  [unwired: 1 in]
                n142 = Subtract(x=w259, y=w257) -> (x-y=w258:cluster{"Numeric":i32, "Numeric":i32})
                n143 = case shown="True" "random position" {
                  tunnel: [w274 w280] -> w265
                  tunnel: w258 -> [_ w276]
                  tunnel: w257 -> [_ w275]
                  frame False {
                    n144 = call "replace_position.vi"("Position"=cluster{"x":dbl, "y":dbl, "z":dbl} {"x"=0.0, "y"=0.0, "z"=0.0}) -> ("Spot"=w274:T1)  [unwired: 1 in, 2 out]
                  }
                  frame True {
                    n145 = Random Number (0-1)() -> (number: 0 to 1=w282:dbl)
                    n146 = Random Number (0-1)() -> (number: 0 to 1=w283:dbl)
                    n147 = Bundle("number: 0 to 1"=w283, "number: 0 to 1"=w282) -> (w281:T15)  [unwired: 1 out]
                    n148 = Multiply(x=w281, y=w276) -> (x*y=w278:cluster{dbl, dbl})
                    n149 = Add(x=w278, y=w275) -> (x+y=w277:cluster{dbl, dbl})
                    n150 = call "coords_image_to_real_currentimage.vi"("Position (pixels on image)"=w277) -> ("Position (real coords)"=w279:cluster{dbl, dbl, "Z":dbl})  [unwired: 9 in]
                    n151 = call "replace_position.vi"("Position"=w279) -> ("Spot"=w280:T1)  [unwired: 1 in, 2 out]
                  }
                }
                n152 = Build Array (concatenate)(w269, w265) -> (w270:T1[])
                n153 = Build Array (concatenate)(w267, cluster{i32, "Label.Visible":bool} {0, "Label.Visible"=TRUE}) -> (w271:T9[])
              }
              event "Position": Value Change {
                # "If the position has changed, translate the spots"
                n154 = event-data() -> ("OldVal"=w292:cluster{"x":dbl, "y":dbl, "z":dbl}, "NewVal"=w293:cluster{"x":dbl, "y":dbl, "z":dbl})  [unwired: 5 out]
                n155 = Subtract(x=w293, y=w292) -> (x-y=w291:cluster{"x":dbl, "y":dbl, "z":dbl})
                n156 = for {
                  tunnel: w296 -> [w301] mode=indexing
                  tunnel: w294 -> [w298] mode=indexing
                  tunnel: [w300] -> w295 mode=indexing
                  tunnel: w291 -> [w299]
                  n157 = Unbundle(w298) -> ("Selected"=w297:bool)  [unwired: 1 out]
                  n158 = case shown="True" w297 {
                    tunnel: w301 -> [w302 w307]
                    tunnel: [w302 w306] -> w300
                    tunnel: w299 -> [_ w303]
                    frame False {
                    }
                    frame True {
                      n159 = call "extract_position.vi"("Spot"=w307) -> ("Position"=w304:cluster{"x":dbl, "y":dbl, "z":dbl})
                      n160 = Add(x=w304, y=w303) -> (x+y=w305:cluster{"x":dbl, "y":dbl, "z":dbl})
                      n161 = call "replace_position.vi"("Position"=w305, "Spot in"=w307) -> ("Spot"=w306:T1)  [unwired: 2 out]
                    }
                  }
                }
              }
              event "Size": Value Change {
                # "If we were constraining the aspect ratio, or preventing a divide by zero, the size control on the FP may be incorrect.  We refresh it in here to stop it displaying a wrong value."
                # "If the size has changed, scale the spots"
                n162 = event-data() -> ("OldVal"=w314:cluster{"x":dbl, "y":dbl, "z":dbl}, "NewVal"=w320:cluster{"x":dbl, "y":dbl, "z":dbl})  [unwired: 5 out]
                n163 = Not Equal?(x=w314, y=w320) -> (x != y?=w313:cluster{"x":bool, "y":bool, "z":bool})
                n164 = Divide(x=w320, y=w314) -> (x/y=w319:cluster{"x":dbl, "y":dbl, "z":dbl})
                n165 = Not Equal To 0?(x=w314) -> (x != 0?=w312:cluster{"x":bool, "y":bool, "z":bool})
                n166 = And(x=w313, y=w312) -> (x .and. y?=w311:cluster{"x":bool, "y":bool, "z":bool})
                n167 = Cluster To Array(cluster=w311) -> (array=w318:bool[])
                n168 = Cluster To Array(cluster=w319) -> (array=w317:dbl[])
                n169 = case shown="True" "lock aspect ratio" {
                  tunnel: w318 -> [w326 w343]
                  tunnel: w317 -> [w325 w341]
                  tunnel: [w323 w333] -> w316
                  frame False {
                    # "We are not constraining the aspect ratio here, so just check we're not introducing NAs"
                    n170 = for {
                      tunnel: w326 -> [w332] mode=indexing
                      tunnel: w325 -> [w328] mode=indexing
                      tunnel: [w330] -> w324 mode=indexing
                      n171 = Not A Number/Path/Refnum?(number/path/refnum=w328) -> (NaN/Path/Refnum?=w329:bool)
                      n172 = Compound Arithmetic op=AND(w332, invert w329) -> (w331:bool)
                      n173 = Select(t=w328, s=w331, f=1.0) -> (s? t:f=w330:dbl)
                    }
                    n174 = Array To Cluster(array=w324) -> (cluster=w323:cluster{"[0]":dbl, "[1]":dbl, "[2]":dbl})
                  }
                  frame True {
                    # "Pick the first element that changed and use it.  Also need to make sure (1) an element did change and (2) everything's valid (no divide by zeros)"
                    n175 = Search 1D Array(1D array=w343, element=TRUE) -> (index of element=w340:i32)  [unwired: 1 in]
                    n176 = Index Array(array=w341, index=w340) -> (element=w336:dbl)
                    n177 = Not A Number/Path/Refnum?(number/path/refnum=w336) -> (NaN/Path/Refnum?=w339:bool)
                    n178 = Less Than 0?(x=w340) -> (x < 0?=w338:bool)
                    n179 = Or(x=w339, y=w338) -> (x .or. y?=w337:bool)
                    n180 = Select(t=1.0, s=w337, f=w336) -> (s? t:f=w334:dbl)
                    n181 = Bundle("x"=w334, "x"=w334, "x"=w334) -> (w333:cluster{"x":dbl, "x":dbl, "x":dbl})  [unwired: 1 in]
                  }
                }
                n182 = for {
                  tunnel: w322 -> [w349] mode=indexing
                  tunnel: w309 -> [w346] mode=indexing
                  tunnel: [w348] -> w310 mode=indexing
                  tunnel: w316 -> [w347]
                  tunnel: w321 -> [w344]
                  n183 = Unbundle(w346) -> ("Selected"=w345:bool)  [unwired: 1 out]
                  n184 = case shown="True" w345 {
                    tunnel: w349 -> [w350 w358]
                    tunnel: [w350 w357] -> w348
                    tunnel: w347 -> [_ w356]
                    tunnel: w344 -> [_ w352]
                    frame False {
                    }
                    frame True {
                      n185 = call "extract_position.vi"("Spot"=w358) -> ("Position"=w354:cluster{"x":dbl, "y":dbl, "z":dbl})
                      n186 = Subtract(x=w354, y=w352) -> (x-y=w355:cluster{"x":dbl, "y":dbl, "z":dbl})
                      n187 = Multiply(x=w355, y=w356) -> (x*y=w353:cluster{"x":dbl, dbl, dbl})
                      n188 = Add(x=w352, y=w353) -> (x+y=w351:cluster{"x":dbl, dbl, dbl})
                      n189 = call "replace_position.vi"("Position"=w351, "Spot in"=w358) -> ("Spot"=w357:T1)  [unwired: 2 out]
                    }
                  }
                }
                n190 = call "find_centroid.vi"("Selection and Groups"=w309, "Spots"=w310) -> ("size"=w308:cluster{"x":dbl, "y":dbl, "z":dbl})  [unwired: 2 in, 4 out]
                n191 = local write "Size"(w308) -> ()
              }
              event "Intensity": Value Change {
                # "When  the user changes intensity, scale all the spots selected so the new mean is correct but keep the ratio between the selected spots.\n\nThe exception to this is when the mean intensity is zero, in which case multiplying makes no sense- in that case we just replace with the new value."
                n192 = event-data() -> ("NewVal"=w359:dbl, "OldVal"=w366:dbl)  [unwired: 5 out]
                n193 = Equal To 0?(x=w366) -> (x = 0?=w362:bool)
                n194 = Not A Number/Path/Refnum?(number/path/refnum=w366) -> (NaN/Path/Refnum?=w361:bool)
                n195 = Or(x=w362, y=w361) -> (x .or. y?=w360:bool)
                n196 = Divide(x=w359, y=w366) -> (x/y=w363:dbl)
                n197 = for {
                  tunnel: w367 -> [w372] mode=indexing
                  tunnel: w364 -> [w374] mode=indexing
                  tunnel: [w371] -> w365 mode=indexing
                  tunnel: w363 -> [w370]
                  tunnel: w360 -> [w369]
                  tunnel: w359 -> [w368]
                  n198 = Unbundle(w374) -> ("Selected"=w373:bool)  [unwired: 1 out]
                  n199 = case shown="True" w373 {
                    tunnel: w372 -> [w375 w382]
                    tunnel: [w375 w379] -> w371
                    tunnel: w370 -> [_ w378]
                    tunnel: w369 -> [_ w377]
                    tunnel: w368 -> [_ w376]
                    frame False {
                    }
                    frame True {
                      n200 = Unbundle By Name(w382) -> ("Intensity"=w380:dbl)
                      n201 = case shown="True" w377 {
                        tunnel: [w385 w386] -> w381
                        tunnel: w380 -> [w384 _]
                        tunnel: w378 -> [w383 _]
                        tunnel: w376 -> [_ w386]
                        frame False {
                          n202 = Multiply(x=w384, y=w383) -> (x*y=w385:dbl)
                        }
                        frame True {
                        }
                      }
                      n203 = Bundle By Name(cluster=w382, "Intensity"=w381) -> (w379:T1)
                    }
                  }
                }
              }
              event "phase": Value Change {
                # "When  the user changes phase, translate the phase of all spots selectedd"
                n204 = event-data() -> ("NewVal"=w388:dbl, "OldVal"=w392:dbl)  [unwired: 5 out]
                n205 = Not A Number/Path/Refnum?(number/path/refnum=w392) -> (NaN/Path/Refnum?=w387:bool)
                n206 = Subtract(x=w388, y=w392) -> (x-y=w389:dbl)
                n207 = for {
                  tunnel: w393 -> [w398] mode=indexing
                  tunnel: w390 -> [w400] mode=indexing
                  tunnel: [w397] -> w391 mode=indexing
                  tunnel: w389 -> [w396]
                  tunnel: w387 -> [w395]
                  tunnel: w388 -> [w394]
                  n208 = Unbundle(w400) -> ("Selected"=w399:bool)  [unwired: 1 out]
                  n209 = case shown="False" w399 {
                    tunnel: w398 -> [w401 w408]
                    tunnel: [w401 w405] -> w397
                    tunnel: w396 -> [_ w404]
                    tunnel: w395 -> [_ w403]
                    tunnel: w394 -> [_ w402]
                    frame False {
                    }
                    frame True {
                      n210 = Unbundle By Name(w408) -> ("Phase"=w406:dbl)
                      n211 = case shown="False" w403 {
                        tunnel: [w411 w412] -> w407
                        tunnel: w406 -> [w410 _]
                        tunnel: w404 -> [w409 _]
                        tunnel: w402 -> [_ w412]
                        frame False {
                          n212 = Add(x=w410, y=w409) -> (x+y=w411:dbl)
                        }
                        frame True {
                        }
                      }
                      n213 = Bundle By Name(cluster=w408, "Phase"=w407) -> (w405:T1)
                    }
                  }
                }
              }
              event "Vortex Charge": Value Change {
                # "When  the user changes l, just set all selected spots to have that value of l."
                n214 = event-data() -> ("NewVal"=w413:i8)  [unwired: 6 out]
                n215 = for {
                  tunnel: w416 -> [w419] mode=indexing
                  tunnel: w414 -> [w421] mode=indexing
                  tunnel: [w418] -> w415 mode=indexing
                  tunnel: w413 -> [w417]
                  n216 = Unbundle(w421) -> ("Selected"=w420:bool)  [unwired: 1 out]
                  n217 = case shown="True" w420 {
                    tunnel: w419 -> [w422 w425]
                    tunnel: [w422 w424] -> w418
                    tunnel: w417 -> [_ w423]
                    frame False {
                    }
                    frame True {
                      n218 = Bundle By Name(cluster=w425, "Vortex Charge"=w423) -> (w424:T1)
                    }
                  }
                }
              }
            }
          }
          frame "Spot Shape" {
            # "We update the spot shape tab only when spots have changed OUTSIDE this tab.  This avoids unnecessary jumping about of the tab control."
            n219 = call "find_centroid.vi"("Selection and Groups"=w436, "Spots"=w437) -> ("Mean Values"=w432:T1)  [unwired: 2 in, 4 out]
            n220 = Wait (ms)(milliseconds to wait=u32 10) -> ()  [unwired: 1 out]
            n221 = call "spots_shape.vi"("Selection and Groups"=w436, "Spots"=w437) -> ("Spot Shape"=w439:enum32{"Normal", "Line", "NA", "Mixed"})  [unwired: 7 in]
            n222 = feedback-in #8(w432) -> ()
            n223 = feedback #8() -> (w433:T1)  [unwired: 1 in]
            n224 = Not Equal?(x=w433, y=w432) -> (x != y?=w438:bool)
            n225 = feedback #9() -> (w428:enum32{"Normal", "Line", "NA", "Mixed"})  [unwired: 1 in]
            n226 = feedback #10() -> (w430:T1)  [unwired: 1 in]
            n227 = Not Equal?(x=w430, y=w432) -> (x != y?=w429:bool)
            n228 = case shown="False" w429 {
              tunnel: w439 -> [_ w558]
              tunnel: ["Spot Shape" w558] -> w427
              frame False {
              }
              frame True {
                n229 = local write "Spot Shape"(w558) -> ()
              }
            }
            n230 = feedback-in #9(w427) -> ()
            n231 = Not Equal?(x=w427, y=w428) -> (x != y?=w426:bool)
            n232 = case shown="\"Normal\", Default" w427 {
              tunnel: w437 -> [w443 w460 w486 w556]
              tunnel: w436 -> [w442 w459 w485 w555]
              tunnel: [w442 w458 w483 w555] -> w434
              tunnel: [w441 w457 w484 w556] -> w435
              tunnel: w432 -> [_ w456 w482 _]
              tunnel: w438 -> [_ w455 w481 _]
              tunnel: w426 -> [_ w453 w479 _]
              frame "Normal", Default {
                # "If \"normal\" is selected, don't allow any NA or line-trapping stuff"
                n233 = for {
                  tunnel: w443 -> [w446] mode=indexing
                  tunnel: w442 -> [w445] mode=indexing
                  tunnel: [w447] -> w441 mode=indexing
                  n234 = Unbundle(w445) -> ("Selected"=w444:bool)  [unwired: 1 out]
                  n235 = case shown="True" w444 {
                    tunnel: [w448 w452] -> w447
                    tunnel: w446 -> [w448 w451]
                    frame False {
                    }
                    frame True {
                      n236 = Bundle By Name(cluster=w451, "NA Position"=cluster{"x":dbl, "y":dbl, "r":dbl} {"x"=0.0, "y"=0.0, "r"=1.0} ("x"), "Line Trapping"=T2 {"Vector"={"x"=0.0, "y"=0.0, "z"=0.0}, "Phase Gradient"=0.0}) -> (w452:T1)
                    }
                  }
                }
              }
              frame "Line" {
                # "If it's out of date, update front panel"
                n237 = Or(x=w455, y=w453) -> (x .or. y?=w454:bool)
                n238 = case shown="True" w454 {
                  tunnel: w456 -> [_ w463]
                  frame False {
                  }
                  frame True {
                    n239 = Unbundle By Name(w463) -> ("Line Trapping"=w462:T2)
                    n240 = local write "Line Trapping"(w462) -> ()
                  }
                }
                n241 = event shown="[1] \"Line Trapping\": Value Change" {
                  selector: _ -> [_ _]
                  dyn-events: _ -> [_ _]
                  timeout: 10 -> [_ _]
                  tunnel: w460 -> [w465 w469]
                  tunnel: w459 -> [w464 w467]
                  tunnel: [w465 w468] -> w457
                  tunnel: [w464 w467] -> w458
                  event Timeout {
                    n242 = event-data() -> ()  [unwired: 3 out]
                  }
                  event Value Change {
                    # "If the line vector has changed, update it"
                    n243 = event-data() -> ("NewVal"=w466:T2)  [unwired: 6 out]
                    n244 = for {
                      tunnel: w469 -> [w474] mode=indexing
                      tunnel: w467 -> [w471] mode=indexing
                      tunnel: [w473] -> w468 mode=indexing
                      tunnel: w466 -> [w472]
                      n245 = Unbundle(w471) -> ("Selected"=w470:bool)  [unwired: 1 out]
                      n246 = case shown="True" w470 {
                        tunnel: w474 -> [w475 w477]
                        tunnel: [w475 w478] -> w473
                        tunnel: w472 -> [_ w476]
                        frame False {
                        }
                        frame True {
                          n247 = Bundle By Name(cluster=w477, "Line Trapping"=w476) -> (w478:T1)
                        }
                      }
                    }
                  }
                }
              }
              frame "NA" {
                n248 = Or(x=w479, y=w481) -> (x .or. y?=w480:bool)
                n249 = case shown="True" w480 {
                  tunnel: w482 -> [_ w491]
                  frame False {
                  }
                  frame True {
                    n250 = Unbundle By Name(w491) -> ("NA Position"=w490:cluster{"x":dbl, "y":dbl, "r":dbl})
                    n251 = call "xyz_to_xy.vi"("Position"=w490) -> ("Position (2D)"=w489:cluster{"x":dbl, "y":dbl}, "z"=w488:dbl)  [unwired: 6 out]
                    n252 = local write "Position on back aperture"(w489) -> ()
                    n253 = local write "Radius on back aperture"(w488) -> ()
                  }
                }
                n254 = event shown="[3] \"Scale BA\": Value Change" {
                  selector: _ -> [_ _ _ _]
                  dyn-events: _ -> [_ _ _ _]
                  timeout: 10 -> [_ _ _ _]
                  tunnel: w486 -> [w493 w499 w520 w542]
                  tunnel: w485 -> [w492 w497 w517 w543]
                  tunnel: [w493 w498 w518 w540] -> w484
                  tunnel: [w492 w497 w517 w543] -> w483
                  event Timeout {
                    n255 = event-data() -> ()  [unwired: 3 out]
                  }
                  event "Position on back aperture": Value Change {
                    # "If the position has changed, translate the spots"
                    n256 = event-data() -> ("OldVal"=w495:cluster{"x":dbl, "y":dbl}, "NewVal"=w496:cluster{"x":dbl, "y":dbl})  [unwired: 5 out]
                    n257 = Subtract(x=w496, y=w495) -> (x-y=w494:cluster{"x":dbl, "y":dbl})
                    n258 = for {
                      tunnel: w499 -> [w504] mode=indexing
                      tunnel: w497 -> [w501] mode=indexing
                      tunnel: [w503] -> w498 mode=indexing
                      tunnel: w494 -> [w502]
                      n259 = Unbundle(w501) -> ("Selected"=w500:bool)  [unwired: 1 out]
                      n260 = case shown="True" w500 {
                        tunnel: w504 -> [w505 w507]
                        tunnel: [w505 w508] -> w503
                        tunnel: w502 -> [_ w509]
                        frame False {
                        }
                        frame True {
                          n261 = Unbundle By Name(w507) -> ("NA Position"=w511:cluster{"x":dbl, "y":dbl, "r":dbl})
                          n262 = call "xy_to_xyz.vi"("Position (2D)"=w509) -> ("Position (3D)"=w510:cluster{dbl, dbl, dbl})  [unwired: 1 in, 2 out]
                          n263 = Add(x=w511, y=w510) -> (x+y=w506:cluster{dbl, dbl, dbl})
                          n264 = Bundle By Name(cluster=w507, "NA Position"=w506) -> (w508:T1)
                        }
                      }
                    }
                  }
                  event "Radius on back aperture": Value Change {
                    # "When  the user changes intensity, scale all the spots selected so the new mean is correct but keep the ratio between the selected spots.\n\nThe exception to this is when the mean intensity is zero, in which case multiplying makes no sense- in that case we just replace with the new value."
                    n265 = event-data() -> ("NewVal"=w512:dbl, "OldVal"=w519:dbl)  [unwired: 5 out]
                    n266 = Equal To 0?(x=w519) -> (x = 0?=w515:bool)
                    n267 = Not A Number/Path/Refnum?(number/path/refnum=w519) -> (NaN/Path/Refnum?=w514:bool)
                    n268 = Or(x=w515, y=w514) -> (x .or. y?=w513:bool)
                    n269 = Divide(x=w512, y=w519) -> (x/y=w516:dbl)
                    n270 = for {
                      tunnel: w520 -> [w525] mode=indexing
                      tunnel: w517 -> [w527] mode=indexing
                      tunnel: [w524] -> w518 mode=indexing
                      tunnel: w516 -> [w523]
                      tunnel: w513 -> [w522]
                      tunnel: w512 -> [w521]
                      n271 = Unbundle(w527) -> ("Selected"=w526:bool)  [unwired: 1 out]
                      n272 = case shown="True" w526 {
                        tunnel: w525 -> [w528 w535]
                        tunnel: [w528 w532] -> w524
                        tunnel: w523 -> [_ w531]
                        tunnel: w522 -> [_ w530]
                        tunnel: w521 -> [_ w529]
                        frame False {
                        }
                        frame True {
                          n273 = Unbundle By Name(w535) -> ("NA Position.r"=w533:dbl)
                          n274 = case shown="False" w530 {
                            tunnel: [w538 w539] -> w534
                            tunnel: w533 -> [w537 _]
                            tunnel: w531 -> [w536 _]
                            tunnel: w529 -> [_ w539]
                            frame False {
                              n275 = Multiply(x=w537, y=w536) -> (x*y=w538:dbl)
                            }
                            frame True {
                            }
                          }
                          n276 = Bundle By Name(cluster=w535, "NA Position.r"=w534) -> (w532:T1)
                        }
                      }
                    }
                  }
                  event "Scale BA": Value Change {
                    n277 = event-data() -> ()  [unwired: 7 out]
                    n278 = for {
                      tunnel: w543 -> [w548] mode=indexing
                      tunnel: w542 -> [w546] mode=indexing
                      tunnel: "Scale back aperture" -> [w545]
                      tunnel: [w544] -> w540 mode=indexing
                      n279 = Unbundle(w548) -> ("Selected"=w547:bool)  [unwired: 1 out]
                      n280 = case shown="True" w547 {
                        tunnel: w546 -> [w549 w550]
                        tunnel: w545 -> [_ w553]
                        tunnel: [w549 w551] -> w544
                        frame False {
                        }
                        frame True {
                          n281 = Unbundle By Name(w550) -> ("NA Position"=w554:cluster{"x":dbl, "y":dbl, "r":dbl})
                          n282 = Multiply(x=w553, y=w554) -> (x*y=w552:cluster{"x":dbl, "y":dbl, "r":dbl})
                          n283 = Bundle By Name(cluster=w550, "NA Position"=w552) -> (w551:T1)
                        }
                      }
                    }
                  }
                }
              }
              frame "Mixed" {
              }
            }
            n284 = call "find_centroid.vi"("Selection and Groups"=w434, "Spots"=w435) -> ("Mean Values"=w431:T1)  [unwired: 2 in, 4 out]
            n285 = feedback-in #10(w431) -> ()
          }
          frame "Rotate" {
            w569 = u32 0 items=["Frame", "Fill", "Highlight"] ("Drawing Mode")
            w568 = u32 0 ("Color")
            w565 = i16 100 ("radius")
            # "It's necessary to check this has changed to stop us unintentionally \"spinning\" the spots..."
            # "Draw the centroid as a spot, then a large circle+cross"
            # "It's important that this loop doesn't go too fast- it hogs the CPU.  However, each tab can have a different loop speed."
            n286 = Unbundle By Name(w562) -> ("Position (Image Pixels)"=w578:cluster{"X":dbl, "Y":dbl}, "Previous Position (Image Pixels)"=w577:cluster{"X":dbl, "Y":dbl}, "Dragging"=w579:bool)
            n287 = feedback-in #11(w562) -> ()
            n288 = feedback #11() -> (w563:T8)  [unwired: 1 in]
            n289 = call "find_centroid.vi"("Selection and Groups"=w580, "Spots"=w583) -> ("centroid"=w576:cluster{"x":dbl, "y":dbl, "z":dbl})  [unwired: 2 in, 4 out]
            n290 = Not Equal?(x=w562, y=w563) -> (x != y?=w560:bool)
            n291 = Wait (ms)(milliseconds to wait=u32 10) -> ()  [unwired: 1 out]
            n292 = And(x=w560, y=w579) -> (x .and. y?=w561:bool)
            n293 = call "coords_real_to_image_currentview.vi"("Position (real coords)"=w576) -> ("Position (pixels, relative to the top left of the image)"=w559:cluster{dbl, dbl})  [unwired: 7 in, 1 out]
            n294 = case shown="True" w561 {
              tunnel: w583 -> [w592 w636]
              tunnel: [w594 w635] -> w582
              tunnel: w580 -> [w593 w637]
              tunnel: [w593 w637] -> w581
              tunnel: w576 -> [w591 w628]
              tunnel: w578 -> [_ w627]
              tunnel: w577 -> [_ w626]
              tunnel: w559 -> [_ w625]
              frame False {
                n295 = event shown="[1] Timeout" {
                  selector: _ -> [_ _]
                  dyn-events: _ -> [_ _]
                  timeout: 10 -> [_ _]
                  tunnel: [w607 w624] -> w594
                  tunnel: w593 -> [w606 _]
                  tunnel: w592 -> [w605 w624]
                  tunnel: w591 -> [w601 _]
                  event "rotate": Value Change {
                    n296 = event-data() -> ()  [unwired: 6 out]
                    n297 = case shown="3" "Rotation Axis" {
                      tunnel: [cluster{dbl, dbl, dbl} {0.0, 0.0, 1.0} ("Custom Axis") cluster{dbl, dbl, dbl} {1.0, 0.0, 0.0} ("Custom Axis") cluster{dbl, dbl, dbl} {0.0, 1.0, 0.0} ("Custom Axis") "Custom Axis"] -> w602
                      frame 0, Default {
                        # "Z"
                      }
                      frame 1 {
                        # "X"
                      }
                      frame 2 {
                        # "Y"
                      }
                      frame 3 {
                      }
                    }
                    n298 = call "normalise_3d_vector.vi"("Vector"=w602) -> ("Unit Vector"=w604:cluster{dbl, dbl, dbl})  [unwired: 3 out]
                    n299 = Divide(x=6.283185307179586, y=360.0) -> (x/y=w599:dbl)
                    n300 = Multiply(x="Angle (degrees)", y=w599) -> (x*y=w596:dbl)
                    n301 = call "arb_rotation_matrix.vi"("Unit Vector"=w604, "theta"=w596) -> ("Real Matrix"=w608:T16)
                    n302 = for {
                      tunnel: w606 -> [w618] mode=indexing
                      tunnel: w605 -> [w613] mode=indexing
                      tunnel: [w614] -> w607 mode=indexing
                      tunnel: w601 -> [w616]
                      tunnel: w608 -> [w615]
                      n303 = Unbundle(w618) -> ("Selected"=w617:bool)  [unwired: 1 out]
                      n304 = case shown="True" w617 {
                        tunnel: w616 -> [_ w623]
                        tunnel: [w619 w622] -> w614
                        tunnel: w613 -> [w619 w621]
                        tunnel: w615 -> [_ w620]
                        frame False {
                        }
                        frame True {
                          n305 = call "apply_matrix_transformation_to_spots.vi"("Transform centre (i.e. transform about this point)"=w623, "Transformation Matrix (3x3)"=w620, "Spot In"=w621) -> ("Spot Out"=w622:T1)  [unwired: 5 out]
                        }
                      }
                    }
                  }
                  event Timeout {
                    n306 = event-data() -> ()  [unwired: 4 out]
                  }
                }
              }
              frame True {
                # "if the mouse has not moved, stuff will be NaN, so let's make like a leopard and not change our spots"
                # "the magnitude of the change in our direction vector gives the rotation angle in radians"
                # "If it's within 100px of the centroid, pretend the mouse is on the surface of a sphere, and synthesize Z accordingly (z^2=100^2-x^2-y^2).  This allows rotation in 3d :)  The output should always be a unit vector."
                n307 = Build Array(w627, w626) -> (w642:cluster{"X":dbl, "Y":dbl}[])
                n308 = for {
                  tunnel: w625 -> [w675]
                  tunnel: w642 -> [w671] mode=indexing
                  tunnel: [w661] -> w641 mode=indexing
                  n309 = Subtract(x=w671, y=w675) -> (x-y=w666:cluster{dbl, dbl})
                  n310 = Divide(x=w666, y=100.0 ("x")) -> (x/y=w667:cluster{dbl, dbl})
                  n311 = Square(x=w667) -> (x^2=w674:cluster{dbl, dbl})
                  n312 = Unbundle(w674) -> (w672:dbl, w673:dbl)
                  n313 = Add(x=w672, y=w673) -> (x+y=w663:dbl)
                  n314 = Subtract(x=1.0, y=w663) -> (x-y=w669:dbl)
                  n315 = Square Root(x=w663) -> (sqrt(x)=w664:dbl)
                  n316 = Greater Than 0?(x=w669) -> (x > 0?=w670:bool)
                  n317 = case shown="False" w670 {
                    tunnel: w669 -> [_ w682]
                    tunnel: [0.0 w681] -> w660
                    tunnel: w667 -> [w679 w680]
                    tunnel: w664 -> [w678 _]
                    tunnel: [w677 w680] -> w662
                    frame False {
                      n318 = Divide(x=w679, y=w678) -> (x/y=w677:cluster{dbl, dbl})
                    }
                    frame True {
                      n319 = Square Root(x=w682) -> (sqrt(x)=w681:dbl)
                    }
                  }
                  n320 = call "xy_to_xyz.vi"("z"=w660, "Position (2D)"=w662) -> ("Position (3D)"=w661:cluster{dbl, dbl, dbl})  [unwired: 2 out]
                }
                n321 = Index Array(array=w641) -> (element #1=w640:cluster{dbl, dbl, dbl}, element #2=w631:cluster{dbl, dbl, dbl})  [unwired: 2 in]
                n322 = Add(x=w640, y=w631) -> (x+y=w630:cluster{dbl, dbl, dbl})
                n323 = Subtract(x=w640, y=w631) -> (x-y=w629:cluster{dbl, dbl, dbl})
                n324 = call "cross_product.vi"("b"=w630, "a"=w629) -> ("a cross b"=w639:cluster{dbl, dbl, dbl})
                n325 = call "normalise_3d_vector.vi"("Vector"=w639) -> ("Unit Vector"=w638:cluster{dbl, dbl, dbl})  [unwired: 3 out]
                n326 = call "normalise_3d_vector.vi"("Vector"=w629) -> ("magnitude"=w633:dbl)  [unwired: 3 out]
                n327 = Not Equal To 0?(x=w633) -> (x != 0?=w632:bool)
                n328 = call "arb_rotation_matrix.vi"("Unit Vector"=w638, "theta"=w633) -> ("Real Matrix"=w634:T16)
                n329 = case shown="True" w632 {
                  tunnel: w637 -> [_ w648]
                  tunnel: w636 -> [w643 w647]
                  tunnel: [w643 w646] -> w635
                  tunnel: w634 -> [_ w645]
                  tunnel: w628 -> [_ w644]
                  frame False {
                  }
                  frame True {
                    n330 = for {
                      tunnel: w648 -> [w654] mode=indexing
                      tunnel: w647 -> [w651] mode=indexing
                      tunnel: [w650] -> w646 mode=indexing
                      tunnel: w645 -> [w652]
                      tunnel: w644 -> [w649]
                      n331 = Unbundle(w654) -> ("Selected"=w653:bool)  [unwired: 1 out]
                      n332 = case shown="True" w653 {
                        tunnel: [w655 w658] -> w650
                        tunnel: w651 -> [w655 w659]
                        tunnel: w652 -> [_ w656]
                        tunnel: w649 -> [_ w657]
                        frame False {
                        }
                        frame True {
                          n333 = call "apply_matrix_transformation_to_spots.vi"("Transform centre (i.e. transform about this point)"=w657, "Transformation Matrix (3x3)"=w656, "Spot In"=w659) -> ("Spot Out"=w658:T1)  [unwired: 5 out]
                        }
                      }
                    }
                  }
                }
              }
            }
            n334 = call "coords_real_to_image_currentview.vi"("Position (real coords)"=w576) -> ("Position (pixels, relative to the top left of the image)"=w571:cluster{dbl, dbl}, "z (real coords)"=w575:dbl)  [unwired: 7 in]
            n335 = expression code="z*1e7+20"(w575) -> (w587:dbl)
            n336 = In Range and Coerce(upper limit=100.0, x=w587, lower limit=2.0) -> (coerced(x)=w574:dbl)  [unwired: 1 out]
            n337 = Bundle("upper limit"=w574, "upper limit"=w574) -> (w567:cluster{"upper limit":dbl, "upper limit":dbl})  [unwired: 1 in]
            n338 = call "myoverlay_oval.vi"("Color"=w568, "Drawing Mode"=w569, "Size"=w567, "Centre Position (pixels on image)"=w571) -> ("Overlay Elements Out"=w573:T17[])  [unwired: 5 in]
            n339 = Bundle("radius"=w565, "radius"=w565) -> (w566:cluster{"radius":i16, "radius":i16})  [unwired: 1 in]
            n340 = call "myoverlay_oval.vi"("Color"=w568, "Drawing Mode"=w569, "Size"=w566, "Centre Position (pixels on image)"=w571, "Overlay Elements In"=w573) -> ("Overlay Elements Out"=w572:T17[])  [unwired: 4 in]
            n341 = Multiply(x=w565, y=cluster{dbl, dbl}[] [{0.0, 0.0}, {1.0, 0.0}, {0.0, 0.0}, {0.0, 1.0}, {0.0, 0.0}, {-1.0, 0.0}, {0.0, 0.0}, {0.0, -1.0}, {0.0, 0.0}]) -> (x*y=w584:cluster{dbl, dbl}[])
            n342 = Add(x=w571, y=w584) -> (x+y=w570:cluster{dbl, dbl}[])
            n343 = call "myoverlay_lines.vi"("Color"=w568, "Drawing Mode"=w569, "Line Endpoints"=w570, "Overlay Elements In"=w572) -> ("Overlay Elements Out"=w564:T17[])  [unwired: 5 in]
          }
          frame "Patterns" {
            n344 = event shown="[3] \"Optimise\": Value Change" {
              selector: _ -> [_ _ _ _ _]
              dyn-events: _ -> [_ _ _ _ _]
              timeout: u32 10 ("milliseconds to wait") -> [_ _ _ _ _]
              tunnel: [w701 w731 w735 w738 w749] -> w684
              tunnel: [w700 w732 w734 w741 w750] -> w683
              tunnel: w686 -> [w699 w731 w735 w739 w748]
              tunnel: w685 -> [w698 w732 w734 w741 w750]
              event "Generate": Value Change {
                # "If there were previous spots, centre the pattern on the spots"
                n345 = event-data() -> ()  [unwired: 1 in, 1 out]
                n346 = call "find_centroid.vi"("Selection and Groups"=w698, "Spots"=w699) -> ("size"=w694:cluster{"x":dbl, "y":dbl, "z":dbl}, "centroid"=w690:cluster{"x":dbl, "y":dbl, "z":dbl}, "# selected"=w696:i16)  [unwired: 2 in, 2 out]
                n347 = Greater?(x=w696, y=i16 1) -> (0:w691:bool)
                n348 = case shown="False" w691 {
                  tunnel: w694 -> [_ w717]
                  tunnel: [cluster{"x":dbl, "y":dbl, "z":dbl} {"x"=2e-05, "y"=2e-05, "z"=2e-05} ("size") w717] -> w693
                  frame False {
                  }
                  frame True {
                  }
                }
                n349 = case shown="\"HCP Shack-Hartmann\"" "Pattern" {
                  tunnel: [w719 w722 w728] -> w692
                  tunnel: w693 -> [_ w721 _]
                  frame "Square Shack-Hartmann" {
                    n350 = call "patterns_square_shack_hartmann.vi"("N"="Spots across centre") -> ("Spots"=w719:T1[])
                  }
                  frame "HCP Shack-Hartmann" {
                    n351 = Unbundle By Name(w721) -> ("x"=w720:dbl)
                    n352 = call "pattern_hcp_shack_hartmann.vi"("Width"=w720, "Reference Array?"="Reference Array?", "Fraction of SLM"="Fraction of SLM", "N"="Spots across centre") -> ("Shack-Hartmann Spots"=w722:T1[])  [unwired: 7 in]
                  }
                  frame "Rectangular Grid" {
                    n353 = call "patterns_rectangular_grid.vi"("spacing/m"="spacing/m", "N"="N") -> ("Spots"=w728:T1[])
                  }
                }
                n354 = local write "Generate"(FALSE ("Generate")) -> ()
                n355 = case shown="True" w691 {
                  tunnel: w692 -> [w704 w708]
                  tunnel: w690 -> [_ w710]
                  tunnel: [w704 w706] -> w702
                  frame False {
                  }
                  frame True {
                    n356 = call "find_centroid.vi"("Spots"=w708) -> ("centroid"=w709:cluster{"x":dbl, "y":dbl, "z":dbl}, "# selected"=→"# selected":i16)  [unwired: 3 in, 3 out]
                    n357 = Subtract(x=w710, y=w709) -> (x-y=w707:cluster{"x":dbl, "y":dbl, "z":dbl})
                    n358 = for {
                      tunnel: w708 -> [w713] mode=indexing
                      tunnel: w707 -> [w712]
                      tunnel: [w711] -> w706 mode=indexing
                      n359 = call "extract_position.vi"("Spot"=w713) -> ("Position"=w714:cluster{"x":dbl, "y":dbl, "z":dbl})
                      n360 = Add(x=w714, y=w712) -> (x+y=w715:cluster{"x":dbl, "y":dbl, "z":dbl})
                      n361 = call "replace_position.vi"("Position"=w715, "Spot in"=w713) -> ("Spot"=w711:T1)  [unwired: 2 out]
                    }
                  }
                }
                "Last Pattern" <- w702
                n362 = call "ensure_selection_matches_spots.vi"("Select All (default: no)"=TRUE ("Select All (default: true)"), "Spots"=w702) -> ("Selection and Groups out"=w700:T9[], "Spots (duplicate)"=w701:T1[])  [unwired: 4 in]
              }
              event "Spots across centre", "Fraction of SLM", "Reference Array?", "N", "spacing/m", "Spots across centre": Value Change {
                n363 = event-data() -> ()  [unwired: 1 in, 1 out]
                n364 = local read "Last Pattern"() -> (w730:T1[])
                n365 = Equal?(x=w731, y=w730) -> (x = y?=w729:bool)
                n366 = case shown="True" w729 {
                  selector: w729 -> [_ w733]
                  frame False {
                  }
                  frame True {
                    n367 = property on="Generate" class="Bool (strict)"("Val(Sgnl)"=w733) -> ()  [unwired: 2 in, 2 out]
                  }
                }
              }
              event Timeout {
                n368 = event-data() -> ()  [unwired: 1 in, 1 out]
              }
              event "Optimise": Value Change {
                n369 = event-data() -> ()  [unwired: 1 in, 1 out]
                n370 = for {
                  N: "Iterations" -> [_]
                  tunnel: 203 ("Optimisation Resolution") -> [w745]
                  shift-right: [w746] -> w738
                  shift-left: w739 -> [w747]
                  tunnel: "Fall-off/m" -> [w742]
                  n371 = call "do_gsw_step.vi"("Optimisation Resolution"=w745, "Sinc Zero"=w742, "Spots In"=w747) -> ("non-uniformity"=→"non-uniformity":dbl, "efficiency"=→"efficiency":dbl, "Spots Out"=w746:T1[])  [unwired: 6 in]
                }
              }
              event "Reset Phase/Amplitude": Value Change {
                n372 = event-data() -> ()  [unwired: 1 in, 1 out]
                n373 = for {
                  tunnel: [w753] -> w749 mode=indexing
                  tunnel: w748 -> [w754] mode=indexing
                  n374 = Bundle By Name(cluster=w754, "Phase"=0.0, "Amplitude Correction"=0.0) -> (w753:T1)
                }
              }
            }
          }
          frame "Plugins" {
            # "The local variable ensures the references are  correct when they make it through to the \"close plugins\" block."
            # "This is the error from loading/unloading VIs on the front panel"
            n375 = control-ref of="Plugin Pnl"() -> (w758:refnum<vi>)
            n376 = Wait (ms)(milliseconds to wait=u32 10) -> ()  [unwired: 1 out]
            n377 = feedback #12() -> (w757:T3)
            n378 = feedback #13() -> (w759:errorcluster)
            n379 = event shown="[1] \"Plugin:\": Value Change" {
              selector: _ -> [_ _ _]
              dyn-events: _ -> [_ _ _]
              timeout: 10 -> [_ _ _]
              tunnel: "Abort Plugin" -> [w766 _ _]
              tunnel: "Plugin:" -> [w771 _ w787]
              tunnel: w759 -> [w770 w785 w789]
              tunnel: [w769 w780 w788] -> w760
              tunnel: [w768 w781 w791] -> w756
              tunnel: w757 -> [w772 w782 w790]
              tunnel: w758 -> [_ w783 _]
              event Timeout {
                n380 = event-data() -> ()  [unwired: 1 in, 2 out]
                n381 = Not(x=w766) -> (.not. x?=w767:bool)
                n382 = case shown="True" w767 {
                  tunnel: w772 -> [w774 w779]
                  tunnel: w771 -> [_ w778]
                  tunnel: w770 -> [w773 w777]
                  tunnel: [w773 w776] -> w769
                  tunnel: [w774 w775] -> w768
                  frame False {
                  }
                  frame True {
                    n383 = call "plugins_run.vi"("Error In"=w777, "Plugin Index"=w778, "Plugins In"=w779) -> ("Error Out"=w776:errorcluster, "Plugins"=w775:T3)  [unwired: 7 in]
                  }
                }
              }
              event "Plugin:": Value Change {
                n384 = event-data() -> ("NewVal"=w784:u16)  [unwired: 1 in]
                n385 = call "plugins_switch.vi"("error in"=w785, "Plugin Pnl"=w783, "Plugin Index"=w784, "Plugins In"=w782) -> ("error out"=w780:errorcluster, "Plugins Out"=w781:T3)  [unwired: 4 in]
              }
              event "Abort Plugin": Value Change {
                n386 = event-data() -> ("NewVal"=w786:bool)  [unwired: 1 in]
                n387 = case shown="True" w786 {
                  tunnel: [w793 w798] -> w791
                  tunnel: w790 -> [w793 w797]
                  tunnel: w789 -> [w792 w796]
                  tunnel: [w792 w795] -> w788
                  tunnel: w787 -> [_ w794]
                  frame False {
                  }
                  frame True {
                    n388 = call "plugins_abort.vi"("Error In"=w796, "Plugin Index"=w794, "Plugins In"=w797) -> ("Error Out"=w795:errorcluster, "Plugins Out"=w798:T3)  [unwired: 7 in]
                  }
                }
              }
            }
            n389 = feedback-in #12(w756) -> ()
            n390 = feedback-in #13(w760) -> ()
            n391 = local write "Plugins"(w756) -> ()
          }
          frame "Video" {
            # "All the controls on this tab are in the bottom (camera) loop."
            n392 = Wait (ms)(milliseconds to wait=u32 10) -> ()  [unwired: 1 out]
            n393 = property on="Property Node" class="ImageControl"(reference=w799) -> ("Image Information String"=→"Image Information":string)  [unwired: 1 in, 2 out]
          }
        }
      }
      event "Tab": Value Change {
        w807 = T18 [enum."Video", enum."Particle Tracking"] items=["Current Spot", "Rotate", "Spot Shape", "Patterns", "Plugins", "Video", "Particle Tracking", "Clamping", "Blank"]
        w812 = refnum<vi> refnum  # Image
        # "This allows us to disable custom mouse-handling for certain tabs.  It can also be done from within the \"mouse down\" event case."
        n394 = event-data() -> ("NewVal"=w808:T4)  [unwired: 1 in, 3 out]
        n395 = Equal?(x=w807, y=w808) -> (x = y?=w806:bool[])
        n396 = Or Array Elements(Boolean array=w806) -> (logical OR=w805:bool)
        n397 = Not(x=w805) -> (.not. x?=w804:bool)
        n398 = Select(t=w811, s=w804, f=w812) -> (s? t:f=w813:refnum<vi>)
        n399 = register-events(reference=w815, w813, w812, w812, w812) -> (reference out=w814:refnum<event-registration>)  [unwired: 1 in, 1 out]
      }
      event Menu Selection (User) {
        n400 = event-data() -> ("ItemTag"=w823:string, "MenuRef"=w816:refnum<k9>)  [unwired: 1 in]
        n401 = case shown="Default" w823 {
          tunnel: w827 -> [w831 w841 w850 w864 w883 w887 w890 w897 w904 w906 w909 w938 w964 w985 w996 w1007 w1010 w1012 w1017 w1020]
          tunnel: w826 -> [w830 w840 w849 w873 w882 w886 w888 w895 w903 w905 w908 w937 w963 w984 w995 w1006 w1009 w1013 w1018 w1019]
          tunnel: [w831 w841 w850 w864 w881 w884 w890 w897 w904 w906 w909 w938 w964 w985 w996 w1007 w1010 w1012 w1017 w1020] -> w825
          tunnel: [w830 w840 w849 w873 w880 w885 w889 w896 w902 w907 w910 w937 w963 w984 w995 w1006 w1009 w1013 w1018 w1019] -> w824
          tunnel: [_ _ _ _ TRUE _ _ _ _ _ _ _ _ _ _ _ _ _ _ _] -> w818
          tunnel: w817 -> [_ _ _ _ _ _ _ _ _ _ _ w936 w962 w976 _ _ _ _ _ _]
          tunnel: w816 -> [_ _ _ _ _ _ _ _ _ _ _ w927 w956 w979 w990 w1001 _ _ _ _]
          frame "ToggleSavingData" {
            # "Data is saved from the middle loop: look there for an explanation."
            n402 = local read "Save Video"() -> (w829:bool)
            n403 = Not(x=w829) -> (.not. x?=w828:bool)
            n404 = local write "Save Video"(w828) -> ()
          }
          frame "SaveStateToFile" {
            # "Save the current settings (i.e. the values of all the controls in VIs that have [Red Tweezers Save Settings] in their documentation string) to a file."
            n405 = call "File Dialog"("prompt"="Please select a location to save the settings", "button label"="Save", "default name"="red_tweezers_settings.xml", "pattern (all files)"="*.xml" ("pattern label"), "pattern label"="XML Settings Files") -> ("selected path"=w839:path, "cancelled"=w832:bool)  [unwired: 7 in, 2 out]
            n406 = Not(x=w832) -> (.not. x?=w833:bool)
            n407 = case shown="True" w833 {
              tunnel: w839 -> [_ w843]
              frame False {
              }
              frame True {
                n408 = Path To String(path=w843) -> (string=w842:string)
                n409 = call "settings_save_to_file.vi"("XML File Path"=w843) -> ()  [unwired: 11 in]
                n410 = call "settings_filename_to_registry.vi"("Last Used Settings File"=w842) -> ()  [unwired: 11 in]
              }
            }
          }
          frame "SaveStateToCurrentFile" {
            # "As SaveStateToFile, but using the current file (i.e. Save not Save As...)."
            n411 = global read "red_tweezers_globals_INTERNAL_VOLATILE.vi" "Current Settings File"() -> (w848:path)
            n412 = call <vilib>:"Check if File or Folder Exists.vi"("path"=w848) -> ("file or folder exists?"=w847:bool, "dup path"=w846:path)  [unwired: 8 in, 1 out]
            n413 = case shown="True" w847 {
              selector: w847 -> [_ w861]
              tunnel: w846 -> [_ w862]
              tunnel: [w853 w862] -> w845
              tunnel: [w854 w861] -> w844
              frame False {
                n414 = call "File Dialog3"("prompt"="Please select a location to save the settings", "button label"="Save", "default name"="red_tweezers_settings.xml", "pattern (all files)"="*.xml" ("pattern label"), "pattern label"="XML Settings Files") -> ("selected path"=w853:path, "cancelled"=w860:bool)  [unwired: 7 in, 2 out]
                n415 = Not(x=w860) -> (.not. x?=w854:bool)
              }
              frame True {
              }
            }
            n416 = case shown="True" w844 {
              tunnel: w845 -> [_ w852]
              frame False {
              }
              frame True {
                n417 = Path To String(path=w852) -> (string=w851:string)
                n418 = call "settings_save_to_file.vi"("XML File Path"=w852) -> ()  [unwired: 11 in]
                n419 = call "settings_filename_to_registry.vi"("Last Used Settings File"=w851) -> ()  [unwired: 11 in]
              }
            }
          }
          frame "LoadStateFromFile" {
            # "Load a file, and use it to reset the values of all the front panel controls."
            # "We need to re-run the initialisation stuff in UDP sender after changing settings\n(for example, this synchronises the settings like camera pixel size with the\nrelevant global variable)"
            n420 = call "File Dialog2"("prompt"="Please select a settings file", "button label"="Open", "default name"="red_tweezers_settings.xml", "pattern (all files)"="*.xml" ("pattern label"), "pattern label"="XML Settings Files") -> ("selected path"=w865:path, "cancelled"=w872:bool)  [unwired: 7 in, 2 out]
            n421 = Not(x=w872) -> (.not. x?=w871:bool)
            n422 = case shown="False" w871 {
              selector: w871 -> [w874 w875]
              tunnel: w865 -> [_ w876]
              tunnel: [w874 w875] -> w863
              frame False {
              }
              frame True {
                n423 = call "settings_load_from_file.vi"("XML File Path"=w876) -> ()  [unwired: 9 in, 2 out]
                n424 = Path To String(path=w876) -> (string=w877:string)
                n425 = call "settings_filename_to_registry.vi"("Last Used Settings File"=w877) -> ()  [unwired: 11 in]
              }
            }
            n426 = call "UDP Sender generic_2.vi"("re-initialise"=w863, "Spots"=w864) -> ()  [unwired: 1 in, 1 out]
          }
          frame "Undo" {
            # "This should get the last undo vector and replace the spots with it :)"
            n427 = call "red_tweezers_UNDO.vi"("Selection/Group"=w882, "Undo/Store (store, False)"=TRUE, "Spots"=w883) -> ("Selection/Group Out (Undo only)"=w880:T9[], "Spots Out (Undo only)"=w881:T1[])  [unwired: 7 in]
          }
          frame "Delete" {
            n428 = call "delete_selected_spots.vi"("Selection/Group 3"=w886, "Spots 3"=w887) -> ("Selection/Group 2"=w885:T9[], "Spots 2"=w884:T1[])  [unwired: 4 in]
          }
          frame "SelectAllSpots" {
            n429 = for {
              tunnel: w888 -> [w893] mode=indexing
              tunnel: [w894] -> w889 mode=indexing
              n430 = Unbundle(w893) -> ("Group ID"=w892:i32)  [unwired: 1 out]
              n431 = Bundle(cluster=w893, "Group ID"=w892, "Selected"=TRUE ("Label.Visible")) -> (w894:T9)
            }
          }
          frame "SelectNoSpots" {
            n432 = for {
              tunnel: w895 -> [w900] mode=indexing
              tunnel: [w901] -> w896 mode=indexing
              n433 = Unbundle(w900) -> ("Group ID"=w899:i32)  [unwired: 1 out]
              n434 = Bundle(cluster=w900, "Group ID"=w899, "Selected"=FALSE ("Label.Visible")) -> (w901:T9)
            }
          }
          frame "SelectSpecificSpots" {
            n435 = call "select_by_id.vi"("Selection/Group"=w903, "Spots"=w904) -> ("Selection/Group Out"=w902:T9[])  [unwired: 9 in]
          }
          frame "Group" {
            # "Group the currently selected spots"
            n436 = call "group_selected_spots.vi"("Selection/Group 2"=w905) -> ("Array"=w907:T9[])
          }
          frame "Ungroup" {
            # "Ungroup the currently selected spots"
            n437 = for {
              tunnel: [w914] -> w910 mode=indexing
              tunnel: w908 -> [w913] mode=indexing
              tunnel: 0 -> [w912]
              n438 = Unbundle(w913) -> ("Selected"=w915:bool)  [unwired: 1 out]
              n439 = case shown="False" w915 {
                tunnel: [w916 w919] -> w914
                tunnel: w913 -> [w916 w918]
                tunnel: w912 -> [_ w917]
                frame False {
                }
                frame True {
                  n440 = Unbundle(w918) -> ("Selected"=w920:bool)  [unwired: 1 out]
                  n441 = Bundle(cluster=w918, "Group ID"=w917, "Selected"=w920) -> (w919:T9)
                }
              }
            }
          }
          frame "ZoomIn" {
            w921 = "ZoomToFit" ("item tag")
            # "turn off \"zoom to fit\""
            n442 = property class="ImageControl"(reference=w936) -> (reference out=w930:refnum<vi>, "ZoomSingle"=w935:cluster{"X":sgl, "Y":sgl}, "Image Center Position"=w928:cluster{"X":u32, "Y":u32})  [unwired: 1 in, 1 out]
            n443 = Unbundle(w935) -> ("X"=w933:sgl)  [unwired: 1 out]
            n444 = Round To Nearest(number=w933) -> (nearest integer value=w929:sgl)
            n445 = Greater Than 0?(x=w929) -> (x > 0?=w934:bool)
            n446 = case shown="True" w934 {
              tunnel: w933 -> [w943 w946]
              tunnel: [w942 w944] -> w932
              frame False {
                n447 = Reciprocal(x=w943) -> (1/x=w940:sgl)
                n448 = Round Toward +Infinity(x=w940) -> (ceil(x): smallest int >= x=w941:sgl)
                n449 = Decrement(x=w941) -> (x-1=w939:sgl)
                n450 = Reciprocal(x=w939) -> (1/x=w942:sgl)
              }
              frame True {
                n451 = Round Toward -Infinity(1:w946) -> (0:w945:sgl)
                n452 = Increment(x=w945) -> (x+1=w944:sgl)
              }
            }
            n453 = Bundle(w932, w932) -> (w931:cluster{sgl, sgl})  [unwired: 1 in]
            n454 = property class="ImageControl"(reference=w930, "ZoomSingle"=w931, "Image Center Position"=w928) -> ()  [unwired: 1 in, 2 out]
            n455 = Get Menu Item Info(7:w921, 11:w927) -> (1:w924:bool, 2:w925:string, 3:w926:refnum<k9>, 6:w923:T19)  [unwired: 1 in, 3 out]
            n456 = Set Menu Item Info(4:w923, 6:FALSE ("checked"), 7:w921, 9:w924, 10:w925, 11:w926) -> ()  [unwired: 1 in, 2 out]
          }
          frame "ZoomOut" {
            w950 = "ZoomToFit" ("item tag")
            # "turn off \"zoom to fit\""
            n457 = property class="ImageControl"(reference=w962) -> (reference out=w958:refnum<vi>, "ZoomSingle"=w961:cluster{"X":sgl, "Y":sgl}, "Image Center Position"=w957:cluster{"X":u32, "Y":u32})  [unwired: 1 in, 1 out]
            n458 = Unbundle(w961) -> ("X"=w947:sgl)  [unwired: 1 out]
            n459 = Greater?(x=w947, y=1.0) -> (0:w949:bool)
            n460 = case shown="False" w949 {
              tunnel: w947 -> [w971 w974]
              tunnel: [w970 w972] -> w960
              frame False {
                n461 = Reciprocal(x=w971) -> (1/x=w968:sgl)
                n462 = Add(x=w968, y=sgl 0.01 ("x")) -> (x+y=w966:sgl)
                n463 = Round Toward -Infinity(1:w966) -> (0:w969:sgl)
                n464 = Increment(x=w969) -> (x+1=w967:sgl)
                n465 = Reciprocal(x=w967) -> (1/x=w970:sgl)
              }
              frame True {
                n466 = Round Toward +Infinity(x=w974) -> (ceil(x): smallest int >= x=w973:sgl)
                n467 = Decrement(x=w973) -> (x-1=w972:sgl)
              }
            }
            n468 = Bundle(w960, w960) -> (w959:cluster{sgl, sgl})  [unwired: 1 in]
            n469 = property class="ImageControl"(reference=w958, "ZoomSingle"=w959, "Image Center Position"=w957) -> ()  [unwired: 1 in, 2 out]
            n470 = Get Menu Item Info(7:w950, 11:w956) -> (1:w953:bool, 2:w954:string, 3:w955:refnum<k9>, 6:w952:T19)  [unwired: 1 in, 3 out]
            n471 = Set Menu Item Info(4:w952, 6:FALSE ("checked"), 7:w950, 9:w953, 10:w954, 11:w955) -> ()  [unwired: 1 in, 2 out]
          }
          frame "ZoomToFit" {
            w980 = "ZoomToFit" ("item tag")
            # "and make sure the image obeys the result"
            # "Toggle menu checkmark"
            n472 = Get Menu Item Info(7:w980, 11:w979) -> (1:w978:bool, 2:w982:string, 3:w983:refnum<k9>, 4:w977:bool, 6:w981:T19)  [unwired: 1 in, 2 out]
            n473 = Not(x=w977) -> (.not. x?=w975:bool)
            n474 = Set Menu Item Info(4:w981, 6:w975, 7:w980, 9:w978, 10:w982, 11:w983) -> ()  [unwired: 1 in, 2 out]
            n475 = property class="ImageControl"(reference=w976, "Zoom to Fit Mode"=w975) -> ()  [unwired: 1 in, 2 out]
          }
          frame "ShowGrid" {
            w991 = "ShowGrid" ("item tag")
            # "Toggle menu checkmark"
            n476 = Get Menu Item Info(7:w991, 11:w990) -> (1:w989:bool, 2:w993:string, 3:w994:refnum<k9>, 4:w988:bool, 6:w992:T19)  [unwired: 1 in, 2 out]
            n477 = Not(x=w988) -> (.not. x?=w987:bool)
            n478 = Set Menu Item Info(4:w992, 6:w987, 7:w991, 9:w989, 10:w993, 11:w994) -> ()  [unwired: 1 in, 2 out]
            n479 = call "grid_and_guides.vi"("Boolean"=w987, "Operation"=T13."Set grid visibility") -> ()  [unwired: 9 in, 1 out]
          }
          frame "ShowGuides" {
            w1002 = "ShowGuides" ("item tag")
            # "Toggle menu checkmark"
            n480 = Get Menu Item Info(7:w1002, 11:w1001) -> (1:w1000:bool, 2:w1004:string, 3:w1005:refnum<k9>, 4:w999:bool, 6:w1003:T19)  [unwired: 1 in, 2 out]
            n481 = Not(x=w999) -> (.not. x?=w998:bool)
            n482 = Set Menu Item Info(4:w1003, 6:w998, 7:w1002, 9:w1000, 10:w1004, 11:w1005) -> ()  [unwired: 1 in, 2 out]
            n483 = call "grid_and_guides.vi"("Boolean"=w998, "Operation"=T13."Set guide visibility") -> ()  [unwired: 9 in, 1 out]
          }
          frame "ConfigureGridAndGuides" {
            n484 = call "grid_and_guides.vi"("Operation"=T13."Show front panel") -> ()  [unwired: 10 in, 1 out]
          }
          frame "ShowSettings" {
            n485 = call "UDP Sender generic_2.vi"("Show panel"=TRUE, "Spots"=w1012) -> ()  [unwired: 1 in, 1 out]
          }
          frame "CameraSettings" {
            n486 = global read "red_tweezers_globals_INTERNAL_VOLATILE.vi" "Current Camera VI"() -> (w1015:path)
            n487 = Open VI Reference(vi path=w1015) -> (vi reference=w1014:refnum<vi>)  [unwired: 5 in, 1 out]
            n488 = property class="VI"(reference=w1014, "Front Panel.Open"=TRUE ("Front Panel Window:Open")) -> ()  [unwired: 1 in, 2 out]
          }
          frame Default {
          }
        }
      }
      event Mouse Down? {
        # "We don't process clicks when the user is on the video tab, so that we can set ROIs."
        # "When the mouse button goes down over the image, we save where it went down, etc. and wait to see what happens next.  We also register to be told when the mouse leaves the control, goes up, or moves.  \"click\" or \"drag\" are only detected once the mouse moves or goes up."
        n489 = event-data() -> ("Coords"=w1034:T20, "Button"=w1028:u16, "Mods"=w1038:cluster{"Double Click":bool, "Menu Key":bool}, "PlatMods"=w1037:T21)  [unwired: 1 in]
        n490 = call "mouse_to_image_coords.vi"("Mouse Coords (screen/pane units)"=w1034, "Image Control"=w1029) -> ("Cursor is on Display Area"=w1027:bool, "Mouse Coords (image pixels)"=w1033:cluster{dbl, dbl})  [unwired: 4 in]
        n491 = disable-structure shown="Enabled" {
          disable-tunnel: w1028 -> [w1046 _]
          disable-tunnel: w1027 -> [w1044 w1047]
          disable-tunnel: [w1043 w1047] -> w1023
          frame Enabled {
            n492 = Equal?(x=u16 1, y=w1046) -> (x = y?=w1045:bool)
            n493 = And(x=w1044, y=w1045) -> (x .and. y?=w1043:bool)
          }
          frame Disabled {
            # "use other pane to allow right-clicking on image"
          }
        }
        n494 = local read "Tab"() -> (w1024:T4)
        n495 = Not Equal?(x=w1024, y=T4."Video" ("Tab")) -> (x != y?=w1022:bool)
        n496 = And(x=w1023, y=w1022) -> (x .and. y?=w1021:bool)
        n497 = case shown="False" w1021 {
          tunnel: w1041 -> [w1050 w1061]
          tunnel: [T8 {"Button Down"=FALSE, "Dragging"=FALSE, "Position (Image Pixels)"={"X"=0.0, "Y"=0.0}, "Previous Position (Image Pixels)"={"X"=0.0, "Y"=0.0}, "Button"=0, "Mods"={"Double Click"=FALSE, "Menu Key"=FALSE}, "PlatMods"={"Shift"=FALSE, "Ctrl"=FALSE, "Alt"=FALSE, "Cmd"=FALSE, "Opt"=FALSE}} w1060] -> w1040
          tunnel: [w1050 w1057] -> w1039
          tunnel: w1028 -> [_ w1056]
          tunnel: w1038 -> [_ w1055]
          tunnel: w1037 -> [_ w1054]
          tunnel: w1033 -> [_ w1053]
          tunnel: [FALSE TRUE] -> w1032
          tunnel: w1029 -> [_ w1051]
          frame False {
            # "If the user clicked on a scrollbar, ignore it and let LabVIEW handle it. (this keeps the scrollbars working)"
          }
          frame True {
            w1059 = FALSE  # Dragging
            w1058 = TRUE  # Button Down
            n498 = register-events(reference=w1061, w1051, w1051, w1051, w1051) -> (reference out=w1057:refnum<event-registration>)  [unwired: 1 in, 1 out]
            n499 = Bundle("Button Down"=w1058, "Dragging"=w1059, "Mouse Coords (image pixels)"=w1053, "Mouse Coords (image pixels)"=w1053, "Button"=w1056, "Mods"=w1055, "PlatMods"=w1054) -> (w1060:T22)  [unwired: 1 in]
          }
        }
        n500 = event-data("Discard?"=w1032) -> ()  [unwired: 4 in, 1 out]
      }
      event Mouse Leave {
        w1068 = refnum<vi> refnum  # Dummy
        # "When the mouse leaves, we reset things."
        n501 = event-data() -> ()  [unwired: 1 in, 2 out]
        n502 = register-events(reference=w1069, w1067, w1068, w1068, w1068) -> (reference out=w1066:refnum<event-registration>)  [unwired: 1 in, 1 out]
      }
      event Mouse Up {
        w1088 = refnum<vi> refnum  # Dummy
        # "Double clicking adds a spot at the mouse position."
        # "deregister"
        # "If we get here the mouse has gone down and up again.  If we've not moved in between, we have a Click.\nEither way we're no longer interested in mouse leave/move/up events."
        n503 = event-data() -> ("Mods"=w1074:cluster{"Double Click":bool, "Menu Key":bool})  [unwired: 1 in, 5 out]
        n504 = Unbundle By Name(w1081) -> ("Dragging"=w1090:bool)
        n505 = Unbundle By Name(w1074) -> ("Double Click"=w1073:bool)
        n506 = Not(x=w1090) -> (.not. x?=w1089:bool)
        n507 = Not(x=w1076) -> (.not. x?=w1078:bool)
        n508 = And(x=w1089, y=w1078) -> (x .and. y?=w1079:bool)
        n509 = case shown="True" w1079 {
          tunnel: w1081 -> [_ w1096]
          tunnel: w1083 -> [w1091 w1094]
          tunnel: w1082 -> [w1092 w1098]
          tunnel: [w1092 w1097] -> w1084
          tunnel: w1073 -> [_ w1095]
          tunnel: [w1091 w1093] -> w1072
          frame False {
          }
          frame True {
            n510 = case shown="True" w1095 {
              tunnel: w1098 -> [w1105 w1148]
              tunnel: [w1103 w1155] -> w1097
              tunnel: w1094 -> [w1099 w1156]
              tunnel: w1096 -> [w1102 w1150]
              tunnel: [w1099 w1152] -> w1093
              frame False {
                w1109 = 400.0  # 20^2 px
                # "If the user clicked, determine which spots should be selected: if we've clicked a spot/group then select it.  Shift-clicking toggles selection for that spot, and leaves the rest of the selection unchanged."
                # "check we're close enough"
                # "find closest"
                n511 = Unbundle By Name(w1102) -> ("Position (Image Pixels)"=w1101:cluster{"X":dbl, "Y":dbl}, "PlatMods.Shift"=w1100:bool)
                n512 = for {
                  tunnel: [w1143] -> w1107 mode=indexing
                  tunnel: w1101 -> [w1142]
                  tunnel: w1099 -> [w1141] mode=indexing
                  # "calculate distances between mouse position and spot positions"
                  n513 = call "extract_position.vi"("Spot"=w1141) -> ("Position"=w1140:cluster{"x":dbl, "y":dbl, "z":dbl})
                  n514 = call "coords_real_to_image_currentview.vi"("Position (real coords)"=w1140) -> ("Position (pixels, relative to the top left of the image)"=w1139:cluster{dbl, dbl})  [unwired: 7 in, 1 out]
                  n515 = Subtract(x=w1139, y=w1142) -> (x-y=w1146:cluster{dbl, dbl})
                  n516 = Multiply(x=w1146, y=w1146) -> (x*y=w1145:cluster{dbl, dbl})
                  n517 = Cluster To Array(cluster=w1145) -> (array=w1144:dbl[])
                  n518 = Add Array Elements(numeric array=w1144) -> (sum=w1143:dbl)
                }
                n519 = Array Max & Min(array=w1107) -> (min value=w1108:dbl, min index (indices)=w1104:i32)  [unwired: 2 out]
                n520 = Less Or Equal?(x=w1108, y=w1109) -> (x <= y?=w1106:bool)
                n521 = case shown="True" w1106 {
                  tunnel: w1105 -> [w1110 w1117]
                  tunnel: w1104 -> [_ w1113]
                  tunnel: w1100 -> [_ w1112]
                  tunnel: [w1110 w1111] -> w1103
                  frame False {
                    # "If we didn't click a spot, do nothing."
                  }
                  frame True {
                    # "If the spot is in a group, act on all spots in that group, not just the spot we clicked."
                    # "This case statement toggles the selection of the spot/group we clicked, and leaves other spots unchanged if we're holding shift.  Otherwise, we select the spot/group that was clicked and deselect everything else."
                    n522 = Index Array(array=w1117, index=w1113) -> (element=w1116:T9)
                    n523 = Unbundle(w1116) -> ("Group ID"=w1114:i32)  [unwired: 1 out]
                    n524 = Greater Than 0?(x=w1114) -> (x > 0?=w1115:bool)
                    n525 = for {
                      tunnel: w1117 -> [w1128] mode=indexing
                      tunnel: w1115 -> [w1125]
                      tunnel: w1114 -> [w1123]
                      tunnel: w1113 -> [w1122]
                      tunnel: w1112 -> [w1120]
                      tunnel: [w1118] -> w1111 mode=indexing
                      i -> [w1121]
                      n526 = Unbundle(w1128) -> ("Group ID"=w1124:i32, "Selected"=w1126:bool)
                      n527 = case shown="False" w1125 {
                        tunnel: w1124 -> [_ w1132]
                        tunnel: [w1130 w1134] -> w1119
                        tunnel: w1123 -> [_ w1133]
                        tunnel: w1122 -> [w1131 _]
                        tunnel: w1121 -> [w1129 _]
                        frame False {
                          n528 = Equal?(x=w1129, y=w1131) -> (x = y?=w1130:bool)
                        }
                        frame True {
                          n529 = Equal?(x=w1132, y=w1133) -> (x = y?=w1134:bool)
                        }
                      }
                      n530 = case shown="True" w1120 {
                        tunnel: [w1135 w1137] -> w1127
                        tunnel: w1126 -> [_ w1138]
                        tunnel: w1119 -> [w1135 w1136]
                        frame False {
                        }
                        frame True {
                          n531 = Exclusive Or(1:w1136, 2:w1138) -> (0:w1137:bool)
                        }
                      }
                      n532 = Bundle("Group ID"=w1124, w1127) -> (w1118:cluster{"Group ID":i32, bool})  [unwired: 1 out]
                    }
                  }
                }
              }
              frame True {
                # "convert mouse position to real coords, and add a spot there."
                # "Double-click detected"
                n533 = Unbundle By Name(w1150) -> ("Position (Image Pixels)"=w1149:cluster{"X":dbl, "Y":dbl})
                n534 = for {
                  tunnel: w1148 -> [w1159] mode=indexing
                  tunnel: [w1158] -> w1147 mode=indexing
                  n535 = Bundle(cluster=w1159, "Selected"=FALSE) -> (w1158:T9)  [unwired: 1 in]
                }
                n536 = call "coords_image_to_real_currentimage.vi"("Position (pixels on image)"=w1149) -> ("Position (real coords)"=w1151:cluster{dbl, dbl, "Z":dbl})  [unwired: 9 in]
                n537 = call "replace_position.vi"("Position"=w1151) -> ("Spot"=w1154:T1)  [unwired: 3 in]
                n538 = Build Array (concatenate)(w1156, w1154) -> (w1152:T1[])
                n539 = Build Array (concatenate)(w1147, T9 {"Group ID"=0, "Selected"=TRUE} ("selection_element")) -> (w1155:T9[])
              }
            }
          }
        }
        n540 = register-events(reference=w1086, w1085, w1088, w1088, w1088) -> (reference out=w1087:refnum<event-registration>)  [unwired: 1 in, 1 out]
      }
      event Mouse Move {
        n541 = event-data() -> ("Coords"=w1173:T20)  [unwired: 1 in, 2 out]
        n542 = call "mouse_to_image_coords.vi"("Mouse Coords (screen/pane units)"=w1173, "Image Control"=w1172) -> ("Mouse Coords (image pixels)"=w1163:cluster{dbl, dbl})  [unwired: 4 in, 1 out]
        n543 = Not(x=w1162) -> (.not. x?=w1167:bool)
        n544 = case shown="True" w1167 {
          tunnel: w1165 -> [_ w1185]
          tunnel: w1171 -> [w1178 w1187]
          tunnel: w1170 -> [w1177 w1186]
          tunnel: [w1177 w1186] -> w1168
          tunnel: [w1178 w1188] -> w1169
          tunnel: w1163 -> [_ w1179]
          frame False {
          }
          frame True {
            # "The \"position\" local variable is there just in case we're on the \"current spot\" tab, so that the position updates nicely"
            # "If the user is dragging, translate the spots.\nHolding down shift causes the mouse's motion to be transformed into scaling about the centroid of the spots and rotation about the same point"
            n545 = Unbundle By Name(w1185) -> ("Position (Image Pixels)"=w1180:cluster{"X":dbl, "Y":dbl})
            n546 = call "find_centroid.vi"("Selection and Groups"=w1186, "Spots"=w1187) -> ("centroid"=w1181:cluster{"x":dbl, "y":dbl, "z":dbl})  [unwired: 2 in, 4 out]
            n547 = Unbundle By Name(w1185) -> ("PlatMods.Shift"=w1184:bool)
            n548 = disable-structure shown="Disabled" {
              disable-tunnel: w1181 -> [w1189 _]
              frame Disabled {
                n549 = local write "Position"(w1189) -> ()
              }
              frame Enabled {
              }
            }
            n550 = call "coords_image_to_real_currentimage.vi"("Position (pixels on image)"=w1179) -> ("Position (real coords)"=w1182:cluster{dbl, dbl, "Z":dbl})  [unwired: 9 in]
            n551 = call "coords_image_to_real_currentimage.vi"("Position (pixels on image)"=w1180) -> ("Position (real coords)"=w1183:cluster{dbl, dbl, "Z":dbl})  [unwired: 9 in]
            n552 = case shown="False" w1184 {
              tunnel: [w1195 w1222] -> w1188
              tunnel: w1187 -> [w1194 w1223]
              tunnel: w1186 -> [w1193 w1221]
              tunnel: w1183 -> [w1192 w1208]
              tunnel: w1181 -> [_ w1218]
              tunnel: w1182 -> [w1191 w1209]
              frame False {
                # "this is the displacement of the mouse, since the last iteration, in \"real\" coordinates (NB the conversions go before subtracting, as it may involve adding a constant as well as multiplying, which would confuse things as we're only interested in displacements here."
                n553 = Subtract(x=w1191, y=w1192) -> (x-y=w1190:cluster{dbl, dbl, "Z":dbl})
                n554 = for {
                  tunnel: w1193 -> [w1200] mode=indexing
                  tunnel: w1194 -> [w1198] mode=indexing
                  tunnel: [w1197] -> w1195 mode=indexing
                  tunnel: w1190 -> [w1196]
                  n555 = Unbundle(w1200) -> ("Selected"=w1199:bool)  [unwired: 1 out]
                  n556 = case shown="True" w1199 {
                    tunnel: w1198 -> [w1201 w1205]
                    tunnel: [w1201 w1204] -> w1197
                    tunnel: w1196 -> [_ w1206]
                    frame False {
                      # "otherwise, leave it alone!"
                    }
                    frame True {
                      # "If the spot is selected, move it by the same amount as the mouse"
                      n557 = call "extract_position.vi"("Spot"=w1205) -> ("Position"=w1203:cluster{"x":dbl, "y":dbl, "z":dbl})
                      n558 = Add(x=w1203, y=w1206) -> (x+y=w1202:cluster{dbl, dbl, dbl})
                      n559 = call "replace_position.vi"("Position"=w1202, "Spot in"=w1205) -> ("Spot"=w1204:T1)  [unwired: 2 out]
                    }
                  }
                }
              }
              frame True {
                # "coordinate conversion to find the rotation and scaling done by the mouse, about the centroid of the spots"
                n560 = Subtract(x=w1208, y=w1218) -> (x-y=w1227:cluster{dbl, dbl, dbl})
                n561 = Subtract(x=w1209, y=w1218) -> (x-y=w1226:cluster{dbl, dbl, dbl})
                n562 = Unbundle(w1226) -> (w1212:dbl, w1213:dbl)  [unwired: 1 out]
                n563 = Unbundle(w1227) -> (w1217:dbl, w1216:dbl)  [unwired: 1 out]
                n564 = Re/Im To Polar(2:w1213, 3:w1212) -> (0:w1210:dbl, 1:w1211:dbl)
                n565 = Re/Im To Polar(2:w1216, 3:w1217) -> (0:w1214:dbl, 1:w1215:dbl)
                n566 = Divide(x=w1211, y=w1215) -> (x/y=w1207:dbl)
                n567 = Subtract(x=w1210, y=w1214) -> (x-y=w1219:dbl)
                n568 = Bundle(w1207, w1207, w1207) -> (w1229:cluster{dbl, dbl, dbl})  [unwired: 1 out]
                n569 = call "scale_matrix.vi"("Scale Factors"=w1229) -> ("Scale Matrix"=w1225:T16)
                n570 = call "arb_rotation_matrix.vi"("Unit Vector"=cluster{dbl, dbl, dbl} {0.0, 0.0, 1.0}, "theta"=w1219) -> ("Real Matrix"=w1224:T16)
                n571 = call-poly <vilib>:"A x B.vi"("B"=w1224, "A"=w1225) -> ("A x B"=w1220:T16)  [unwired: 1 out]
                n572 = for {
                  tunnel: w1223 -> [w1235] mode=indexing
                  tunnel: [w1234] -> w1222 mode=indexing
                  tunnel: w1221 -> [w1233] mode=indexing
                  tunnel: w1218 -> [w1231]
                  tunnel: w1220 -> [w1230]
                  n573 = Unbundle(w1233) -> ("Selected"=w1232:bool)  [unwired: 1 out]
                  n574 = case shown="True" w1232 {
                    tunnel: w1235 -> [w1236 w1240]
                    tunnel: [w1236 w1239] -> w1234
                    tunnel: w1231 -> [_ w1238]
                    tunnel: w1230 -> [_ w1237]
                    frame False {
                    }
                    frame True {
                      n575 = call "apply_matrix_transformation_to_spots.vi"("Transform centre (i.e. transform about this point)"=w1238, "Transformation Matrix (3x3)"=w1237, "Spot In"=w1240) -> ("Spot Out"=w1239:T1)  [unwired: 5 out]
                    }
                  }
                }
              }
            }
          }
        }
        n576 = Unbundle By Name(w1165) -> ("Position (Image Pixels)"=w1164:cluster{"X":dbl, "Y":dbl})
        n577 = Bundle By Name(cluster=w1165, "Dragging"=TRUE, "Previous Position (Image Pixels)"=w1164, "Position (Image Pixels)"=w1163) -> (w1175:T8)
      }
      event "stop": Value Change {
        n578 = event-data() -> ()  [unwired: 1 in, 4 out]
        n579 = global read "red_tweezers_globals_INTERNAL_VOLATILE.vi" "Current Settings File"() -> (w1244:path)
        n580 = call <vilib>:"Check if File or Folder Exists.vi"("path"=w1244) -> ("file or folder exists?"=w1243:bool)  [unwired: 8 in, 2 out]
        n581 = case shown="False" w1243 {
          tunnel: [w1251 w1255] -> w1245
          frame False {
            n582 = Two Button Dialog(message="Save current settings?", 1:"Don't Save" ("F button name (\"Cancel\")"), 2:"Save As..." ("T button name (\"OK\")")) -> (T button?=w1248:bool)
            n583 = Select(t=T14."Center Button" ("Which Button?"), s=w1248, f=T14."Right Button" ("Which Button?")) -> (s? t:f=w1251:T14)
          }
          frame True {
            n584 = call <vilib>:"Three Button Dialog.vi"("Allow user to close window? (TRUE)"=TRUE, "Window Title (\"\")"="Save Settings?" ("Window Title (\"\")"), "Right Button Text (\"Cancel\")"="No" ("Right Button Text (\"Cancel\")"), "Center Button Text (\"No\")"="Save As..." ("Center Button Text (\"No\")"), "Left Button Text (\"Yes\")"="Save" ("Left Button Text (\"Yes\")"), "message"="Would you like to save the current settings? You can choose to use the current settings file or save to a new location.") -> ("Which Button?"=w1255:T14)  [unwired: 5 in]
          }
        }
        n585 = case shown="\"Center Button\"" w1245 {
          tunnel: [TRUE TRUE FALSE FALSE] -> w1242
          frame "Left Button", Default {
          }
          frame "Center Button" {
            n586 = call "File Dialog5"("prompt"="Please select a location to save the settings", "button label"="Save", "default name"="red_tweezers_settings.xml", "pattern (all files)"="*.xml" ("pattern label"), "pattern label"="XML Settings Files") -> ("selected path"=w1263:path)  [unwired: 7 in, 3 out]
            n587 = global write "red_tweezers_globals_INTERNAL_VOLATILE.vi" "Current Settings File"(w1263) -> ()
          }
          frame "Right Button" {
          }
          frame "Window Close" {
          }
        }
        n588 = global write "red_tweezers_globals_INTERNAL_VOLATILE.vi" "Save Settings On Exit"(w1242) -> ()
      }
    }
    n589 = case shown="True" w192 {
      tunnel: w198 -> [_ w215]
      frame False {
      }
      frame True {
        n590 = global write "red_tweezers_globals_INTERNAL.vi" "Image Overlay (extras from control loop)"(w215) -> ()
      }
    }
    n591 = call "red_tweezers_UNDO.vi"("Force Save"=w194, "This change is inconsequential (don't save it)"=w195, "Selection/Group"=w196, "Spots"=w197) -> ()  [unwired: 6 in, 2 out]
    n592 = call "sync_with_globals.vi"("Selection/Group"=w196, "Spots"=w197) -> ("Selection/Group 2"=w208:T9[], "Spots 2"=w190:T1[])  [unwired: 4 in]
    n593 = feedback #14() -> (w213:T11)  [unwired: 1 out]
    n594 = call "Smoothed Frame Rate.vi"("Feedback In"=w213) -> ("Feedback Out"=w212:T11, "Frame Rate"=→"Interface Frame Rate":dbl)  [unwired: 1 in, 4 out]
    n595 = feedback-in #14(w212) -> ()
    n596 = case shown="False" w189 {
      tunnel: w190 -> [w1272 _]
      frame False {
        n597 = call "UDP Sender generic_2.vi"("Spots"=w1272) -> ()  [unwired: 2 in, 1 out]
      }
      frame True {
      }
    }
  }
  n598 = while {
    tunnel: w8 -> [w1290]
    shift-right: [w1289] -> w7
    shift-left: w9 -> [w1291]
    shift-right: [w1286] -> _
    shift-left: _ -> [w1279]
    shift-right: [w1285] -> _
    shift-left: _ -> [w1283]
    shift-right: [w1284] -> _
    shift-left: FALSE ("Saving") -> [w1280]
    stop <- w1288 stop-if-true
    w1277 = u32 50 ("millisecond multiple")
    # "Start/stop saving data, if necessary"
    n599 = Divide(x=u32 1000, y=w1277) -> (x/y=w1275:dbl)
    n600 = Wait Until Next ms Multiple(millisecond multiple=w1277) -> ()  [unwired: 1 out]
    n601 = call "imageQ_dequeue.vi"("timeout in ms (-1)"=2000, "Return queue"=w1291, "Image Dst"=w1290) -> ("Timestamp/us"=w1281:u64, "Return queue out"=w1289:refnum<queue>, "Image Dst Out"=w1292:T7, "timed out?"=w1295:bool, "ROI"=w1274:u64[])  [unwired: 4 in]
    n602 = Not(x=w1295) -> (.not. x?=w1293:bool)
    n603 = case shown="True" w1293 {
      tunnel: w1292 -> [_ w1328]
      tunnel: w1283 -> [w1322 w1331]
      tunnel: w1280 -> [_ w1325]
      tunnel: [w1322 w1326] -> w1282
      tunnel: w1281 -> [_ w1329]
      tunnel: w1279 -> [w1323 w1330]
      tunnel: [w1323 w1327] -> w1278
      tunnel: w1274 -> [_ w1324]
      frame False {
      }
      frame True {
        n604 = global read "red_tweezers_globals_INTERNAL.vi" "Image Overlay (extras from control loop)"() -> (w1340:T17[])
        n605 = case shown="True" w1325 {
          tunnel: w1331 -> [w1341 w1343]
          tunnel: w1330 -> [w1342 w1349]
          tunnel: w1329 -> [_ w1348]
          tunnel: w1328 -> [_ w1347]
          tunnel: [w1342 w1346] -> w1327
          tunnel: [w1341 w1345] -> w1326
          frame False {
          }
          frame True {
            n606 = call "save_data_save.vi"("Image"=w1347, "Timestamp"=w1348, "Avi Refnum"=w1343, "Data refnum"=w1349) -> ("error out"=w1344:errorcluster, "Avi Refnum (duplicate)"=w1345:T23, "Data refnum (duplicate)"=w1346:refnum<file>)  [unwired: 5 in]
            n607 = case shown="Error" w1344 {
              selector: w1344 -> [_ w1351]
              frame No Error {
              }
              frame Error {
                n608 = call <vilib>:"Clear Errors.vi"("error in (no error)"=w1351) -> ()  [unwired: 6 in, 1 out]
                n609 = local write "Save Video"(FALSE ("Save")) -> ()
              }
            }
          }
        }
        n610 = global write "red_tweezers_globals_INTERNAL.vi" "Global ROI"(w1324) -> ()
        n611 = global read "red_tweezers_globals_INTERNAL_VOLATILE.vi" "Tracked Spot Positions (3D)"() -> (w1332:cluster{"x":dbl, "y":dbl, "Z":dbl}[])
        n612 = global read "red_tweezers_globals.vi" "Selection/Group"() -> (w1339:T9[])
        n613 = global read "red_tweezers_globals.vi" "Spots"() -> (w1338:T1[])
        n614 = call "overlay_positions.vi"("Positions"=w1332, "Image"=w1328) -> ("Image 2"=w1334:T7)  [unwired: 9 in]
        n615 = call "render_overlay_elements.vi"("Image Overlay (extras from control loop)"=w1340, "Image"=w1334) -> ("Image Out"=w1337:T7)  [unwired: 5 in]
        n616 = call "grid_and_guides.vi"("Operation"=T13."Render on image", "Image"=w1337) -> ("Image Out"=w1335:T7)  [unwired: 9 in]
        n617 = call "overlay_spots_on_image.vi"("Selection and Groups"=w1339, "Spots"=w1338, "image"=w1335) -> ("Image"=→"Image":T7)  [unwired: 3 in, 1 out]
      }
    }
    n618 = global read "red_tweezers_globals_INTERNAL_VOLATILE.vi" "Video Frame Rate"() -> (→"Video Frame Rate":dbl)
    n619 = case shown="True" "Save Video" {
      tunnel: [w1298 w1313] -> w1286
      tunnel: [w1297 w1307] -> w1285
      tunnel: [FALSE ("Saving") w1312] -> w1284
      tunnel: w1280 -> [w1301 w1311]
      tunnel: w1282 -> [w1299 w1310]
      tunnel: w1278 -> [w1300 w1309]
      tunnel: w1275 -> [_ w1308]
      frame False {
        n620 = case shown="True" w1301 {
          tunnel: w1300 -> [w1303 w1306]
          tunnel: w1299 -> [w1302 w1305]
          tunnel: [w1303 _] -> w1298
          tunnel: [w1302 _] -> w1297
          frame False {
          }
          frame True {
            n621 = local write "Save Video"(FALSE ("Save")) -> ()
            n622 = call "save_data_stop.vi"("Avi Refnum"=w1305, "Data refnum"=w1306) -> ()  [unwired: 10 in]
          }
        }
      }
      frame True {
        n623 = case shown="False" w1311 {
          selector: w1311 -> [_ w1321]
          tunnel: [w1318 w1319] -> w1313
          tunnel: [w1317 w1320] -> w1307
          tunnel: [w1314 w1321] -> w1312
          tunnel: w1310 -> [_ w1320]
          tunnel: w1309 -> [_ w1319]
          tunnel: w1308 -> [w1316 _]
          frame False {
            n624 = call "save_data_start.vi"("Save Video"=TRUE, "Frames Per Second"=w1316) -> ("Saving"=w1314:bool, "Avi Refnum"=w1317:T23, "Data Refnum"=w1318:refnum<file>)  [unwired: 3 in]
            n625 = local write "Save Video"(w1314) -> ()
          }
          frame True {
          }
        }
      }
    }
    n626 = local read "stop"() -> (w1288:bool)
  }
  n627 = Release Queue(queue=w7) -> ()  [unwired: 2 in, 3 out]
  n628 = case shown="True" w1 {
    frame False {
    }
    frame True {
      n629 = One Button Dialog(message="Warning: there was a camera error.  You may need to restart Red Tweezers.") -> ()  [unwired: 1 in, 1 out]
    }
  }
  n630 = flat-sequence {
    tunnel: w17 -> [w1357]
    tunnel: w16 -> [_]
    frame #0 {
      # "This autosaves when we stop.  The sequence structures are necessary so that:\n1. loading settings doesn't stop the VI\n2. plugins are still open (and hence saved) when we save settings"
      n631 = local read "Plugins"() -> (w1360:T3)
      n632 = global read "red_tweezers_globals_INTERNAL_VOLATILE.vi" "Current Settings File"() -> (w1354:path)
      n633 = global read "red_tweezers_globals_INTERNAL_VOLATILE.vi" "Save Settings On Exit"() -> (w1353:bool)
      n634 = flat-sequence {
        tunnel: w1357 -> [w1363]
        tunnel: [w1363] -> w1356
        frame #0 {
          n635 = local write "stop"(FALSE ("STOP")) -> ()
        }
      }
      n636 = case shown="True" w1353 {
        tunnel: w1354 -> [_ w1368]
        tunnel: w1356 -> [w1365 w1366]
        tunnel: [w1365 w1366] -> w1355
        frame False {
        }
        frame True {
          n637 = Path To String(path=w1368) -> (string=w1367:string)
          n638 = call "settings_save_to_file.vi"("XML File Path"=w1368) -> ()  [unwired: 11 in]
          n639 = call "settings_filename_to_registry.vi"("Last Used Settings File"=w1367) -> ()  [unwired: 11 in]
        }
      }
      n640 = flat-sequence {
        tunnel: w1355 -> [w1361]
        tunnel: [w1361] -> _
        frame #0 {
          n641 = local write "stop"(TRUE ("STOP")) -> ()
        }
      }
      n642 = control-ref of="Plugin Pnl"() -> (w1358:refnum<vi>)
      n643 = control-ref of="Plugin:"() -> (w1359:refnum<vi>)
      n644 = call "plugins_unload.vi"("error in (no error)"=w1355, "Plugins"=w1360, "Sub Panel"=w1358, "Plugin Chooser"=w1359) -> ()  [unwired: 2 in, 2 out]
    }
  }
